vi "fpga_main.vi"() -> ()   [LabVIEW 2013]
uses:
  <vilib>/rvi/FXPMathLib/FxpDiv/subVIs/nifxpmath_Div_SimConfig.ctl
  <vilib>/rvi/Emulation/niFpgaSctlEmulationGetInTimedLoop.vi
  <vilib>/rvi/eio/common/nirviEmuTemplateMethod_errors.vi
  <vilib>/rvi/Emulation/niFpgaProcessEmulError.vi
  <vilib>/rvi/Emulation/niFpgaEmulationReportErrorSimple.vi
  <vilib>/rvi/Emulation/niFpgaGetClockAttributes.vi
  <vilib>/rvi/FXPMathLib/FxpDiv/simVIs/DllFxpDivTemp_sub.vi
  <vilib>/rvi/Emulation/niFpgaCriticalErrorInLSC.vi
  <vilib>/rvi/interface/RandomDataEmulation/nirviRandomDataFPGAFIFO.vi
  <vilib>/rvi/interface/RandomDataEmulation/niFpgaRandomDataHandleErrors.vi
  <vilib>/eio/EIONode/EIONode.xnode
  <vilib>/rvi/FXPMathLib/FxpDiv/XNode/nifxpmath_Div.xnode
  <vilib>/rvi/FXPMathLib/FxpMul/XNode/nifxpmath_Multiplier.xnode
  <vilib>/rvi/FXPMathLib/FxpSub/XNode/nifxpmath_Sub.xnode
  <vilib>/rvi/FXPMathLib/FxpAdd/XNode/nifxpmath_Add.xnode
  <vilib>/rvi/DataTransferAndStorage/Container/XNode/niFpgaContainer.xnode
  <vilib>/rvi/interface/RandomDataEmulation/nirviRandomDataFpgaReadWriteTemplate.vi
  <vilib>/rvi/FXPMathLib/sim/FxpSim.dll
panel:
  out "CoinToss":bool
  out "AutoDispense 4":bool
  out "AutoDispense 3":bool
  out "AutoDispense 1":bool
  out "AutoDispense 2":bool
  out "SensorOffset 4":bool
  out "SensorOffset 3":bool
  out "SensorOffset 2":bool
  out "SensorOffset 1":bool
  in  "Opto On Time 1 (mSec)":u32=5000
  out "Opto Rand Pre":bool
  out "OptoPre 4":bool
  out "OptoPre 3":bool
  out "OptoPre 2":bool
  out "npcountout 4":i16
  in  "npcountin 4":i16
  out "npcountout 3":i16
  in  "npcountin 3":i16
  out "npcountout 2":i16
  in  "npcountin 2":i16
  out "npcountout":i16
  in  "npcountin":i16
  out "angle_out 4":bool
  out "angle_out 3":bool
  out "angle_out 2":bool
  out "angle_out 1":bool
  out "Contingency 4":bool
  out "AI9":fxp<+/-,24,5>
  out "AI8":fxp<+/-,24,5>
  out "Contingency 3":bool
  out "AI6":fxp<+/-,24,5>
  out "AI5":fxp<+/-,24,5>
  out "Contingency 2":bool
  out "AI4":fxp<+/-,24,5>
  out "AI3":fxp<+/-,24,5>
  out "Contingency 1":bool
  out "AI1":fxp<+/-,24,5>
  out "AI2":fxp<+/-,24,5>
  out "flashdisp 4":bool
  out "flashdisp 3":bool
  out "flashdisp 2":bool
  out "flashdisp 1":bool
  out "Automatic Dispense Trigger 4":bool
  out "Automatic Dispense Trigger 3":bool
  in  "Trial Live In 1":bool
  in  "Hold In 1":bool
  in  "Hold Count In 1":i16 format="%.0g"
  out "TurnOnOpto 1":bool
  out "Dispense Trigger 1":bool
  in  "Trial Live In 4":bool
  in  "Hold In 4":bool
  in  "Hold Count In 4":i16 format="%.0g"
  out "TurnOnOpto 4":bool
  out "Opto Rand Met 1":bool
  out "Opto Rand Met 4":bool
  out "Dispense Trigger 4":bool
  in  "Trial Live In 3":bool
  in  "Hold In 3":bool
  in  "Hold Count In 3":i16 format="%.0g"
  in  "Trial Live In 2":bool
  in  "Hold In 2":bool
  in  "Hold Count In 2":i16 format="%.0g"
  out "Opto Rand Met 3":bool
  out "Opto Rand Met 2":bool
  out "TurnOnOpto 3":bool
  out "TurnOnOpto 2":bool
  out "Automatic Dispense Trigger 2":bool
  out "Dispense Trigger 3":bool
  out "Dispense Trigger 2":bool
  out "Automatic Dispense Trigger 1":bool
  in  "Tab Control":T1(tab)
  in  "Automated Pellets Target 1":u16=200
  in  "X Center 1":fxp<+/-,24,5>
  in  "Y Center 1":fxp<+/-,24,5>
  in  "Radius Voltage 1":fxp<+/-,24,5>=1.0
  out "Touch 1 1":bool
  out "Touch 2 1":bool
  out "Nose Poke 1":bool
  out "X 1":fxp<+/-,22,10> format="%.16g"
  out "Y 1":fxp<+/-,22,10> format="%.16g"
  in  "Inner Threshold 1":fxp<+,22,9>=100.0 format="%.23g"
  in  "Hold Duration 1":i16=50
  out "Trial Live 1":bool
  out "Hold 1":bool
  out "Hold Count 1":i16 format="%.0g"
  out "Deviation 1":fxp<+,22,10> format="%.16g"
  in  "Sequence Override 1":bool
  in  "OptoEnable 1":bool
  out "Automated Pellets Dispensed 1":u16
  out "Pellets Dispensed 1":u16
  out "Dispense 1":bool
  in  "Automatic Dispense 1":bool
  in  "Mean 1":fxp<+,22,9>=100.0
  in  "Opto Chance 1 %":fxp<+,16,8>=50.0
  out "Lick 1":bool
  in  "Override Fail when moved out":bool
  in  "Dispense time 1":u32=100
  out "angle":fxp<+/-,9,9>
  in  "Flip 1 1":bool
  in  "Flip 2 1":bool
  in  "Flip XY 1":bool
  in  "Outer\nThreshold 1":fxp<+,22,9>=1.0
  in  "Min Angle 1":fxp<+,9,9> format="%.52g"
  in  "Max Angle 1":fxp<+,9,9>=360.0 format="%.52g"
  in  "Override Approach 1":bool
  in  "Opto on 1":bool
  in  "CCW(T) 1":bool
  in  "Min Angle 1 2":fxp<+,9,9> format="%.52g"
  in  "Max Angle 1 2":fxp<+,9,9>=360.0 format="%.52g"
  in  "CCW(T) 1 2":bool
  in  "Opto OnPost Time 1 (mSec)":u32=5000
  in  "Opto on 2":bool
  out "Deviation 2":fxp<+,22,10> format="%.16g"
  in  "Inner Threshold 2":fxp<+,22,9>=100.0 format="%.23g"
  in  "Hold Duration 2":i16=50
  out "Trial Live 2":bool
  out "Hold 2":bool
  out "Hold Count 2":i16 format="%.0g"
  out "Automated Pellets Dispensed 2":u16
  in  "Automated Pellets Target 2":u16
  out "Pellets Dispensed 2":u16
  in  "Automatic Dispense 2":bool
  in  "Mean 2":fxp<+,22,9>=100.0
  out "Dispense 2":bool
  out "Y 2":fxp<+/-,22,10> format="%.16g"
  out "X 2":fxp<+/-,22,10> format="%.16g"
  out "Nose Poke 2":bool
  out "Touch 2 2":bool
  out "Touch 1 2":bool
  in  "Radius Voltage 2":fxp<+/-,24,5>=1.0
  in  "Flip XY 2":bool
  in  "Flip 2 2":bool
  in  "Flip 1 2":bool
  in  "Outer\nThreshold 2":fxp<+,22,9>=1.0
  in  "Y Center 2":fxp<+/-,24,5>
  in  "X Center 2":fxp<+/-,24,5>
  in  "Sequence Override 2":bool
  in  "OptoEnable 2":bool
  in  "Opto Chance 2 %":fxp<+,16,8>=50.0
  out "Lick 2":bool
  in  "Override Fail when moved out 2":bool
  in  "Dispense time 2":u32=100
  out "angle 2":fxp<+/-,9,9>
  in  "Opto On Time 2 (mSec)":u32=5000
  in  "Override Approach 2":bool
  in  "Min Angle 2":fxp<+,9,9> format="%.52g"
  in  "Max Angle 2":fxp<+,9,9>=360.0 format="%.52g"
  in  "CCW(T)  2":bool
  in  "CCW(T)  2 2":bool
  in  "Min Angle 2 2":fxp<+,9,9> format="%.52g"
  in  "Max Angle 2 2":fxp<+,9,9>=360.0 format="%.52g"
  in  "Opto OnPost Time 2 (mSec)":u32=5000
  out "Deviation 3":fxp<+,22,10> format="%.16g"
  in  "Inner Threshold 3":fxp<+,22,9>=100.0 format="%.23g"
  in  "Hold Duration 3":i16=50
  out "Hold 3":bool
  out "Hold Count 3":i16 format="%.0g"
  out "Trial Live 3":bool
  out "Y 3":fxp<+/-,22,10> format="%.16g"
  out "X 3":fxp<+/-,22,10> format="%.16g"
  out "Nose Poke 3":bool
  out "Touch 2 3":bool
  out "Touch 1 3":bool
  in  "Radius Voltage 3":fxp<+/-,24,5>=1.0
  in  "Flip XY 3":bool
  in  "Flip 2 3":bool
  in  "Flip 1 3":bool
  in  "Outer\nThreshold 3":fxp<+,22,9>=1.0
  in  "Y Center 3":fxp<+/-,24,5>
  in  "X Center 3":fxp<+/-,24,5>
  out "Dispense 3":bool
  in  "Automatic Dispense 3":bool
  in  "Mean 3":fxp<+,22,9>=100.0
  out "Pellets Dispensed 3":u16
  in  "Automated Pellets Target 3":u16
  out "Automated Pellets Dispensed 3":u16
  in  "Sequence Override 3":bool
  in  "OptoEnable 3":bool
  in  "Opto On Time 3(mSec)":u32=5000 caption="Opto On Time 3 (mSec)"
  in  "Opto Chance 3 %":fxp<+,16,8>=50.0
  out "Lick 3":bool
  in  "Override Fail when moved out 3":bool
  in  "Dispense time 3":u32=100
  out "angle 3":fxp<+/-,9,9>
  in  "Override Approach 3":bool
  in  "Opto on 3":bool
  in  "Min Angle 3":fxp<+,9,9> format="%.52g"
  in  "Max Angle 3":fxp<+,9,9>=360.0 format="%.52g"
  in  "CCW(T)  3":bool
  in  "Min Angle 3 2":fxp<+,9,9> format="%.52g"
  in  "Max Angle 3 2":fxp<+,9,9>=360.0 format="%.52g"
  in  "CCW(T)  3 2":bool
  in  "Opto OnPost Time 3 (mSec)":u32=5000
  in  "Opto On Time 4 (mSec)":u32=5000
  in  "X Center 4":fxp<+/-,24,5>
  in  "Y Center 4":fxp<+/-,24,5>
  in  "Outer\nThreshold 4":fxp<+,22,9>=1.0
  in  "Flip 1 4":bool
  in  "Flip 2 4":bool
  in  "Flip XY 4":bool
  in  "Radius Voltage 4":fxp<+/-,24,5>=1.0
  out "Touch 1 4":bool
  out "Touch 2 4":bool
  out "Nose Poke 4":bool
  out "X 4":fxp<+/-,22,10> format="%.16g"
  out "Y 4":fxp<+/-,22,10> format="%.16g"
  in  "Inner Threshold 4":fxp<+,22,9>=100.0 format="%.23g"
  in  "Hold Duration 4":i16=50
  out "Hold 4":bool
  out "Hold Count 4":i16 format="%.0g"
  out "Trial Live 4":bool
  out "Deviation 4":fxp<+,22,10> format="%.16g"
  in  "Sequence Override 4":bool
  in  "OptoEnable 4":bool
  out "Automated Pellets Dispensed 4":u16
  out "Pellets Dispensed 4":u16
  in  "Automated Pellets Target 4":u16
  out "Dispense 4":bool
  in  "Automatic Dispense 4":bool
  in  "Mean 4":fxp<+,22,9>=100.0
  in  "Opto Chance 4 %":fxp<+,16,8>=50.0
  out "Lick 4":bool
  in  "Override Fail when moved out 4":bool
  in  "Dispense time 4":u32=100
  out "angle 4":fxp<+/-,9,9>
  in  "Override Approach 4":bool
  in  "Opto on 4":bool
  in  "Min Angle 4":fxp<+,9,9> format="%.52g"
  in  "Max Angle 4":fxp<+,9,9>=360.0 format="%.52g"
  in  "CCW(T)  4":bool
  in  "Min Angle 4 2":fxp<+,9,9> format="%.52g"
  in  "Max Angle 4 2":fxp<+,9,9>=360.0 format="%.52g"
  in  "CCW(T)  4 2":bool
  in  "Opto OnPost Time 4 (mSec)":u32=5000
  in  "Opto Current 2 (mA)":fxp<+/-,16,8>=65.0
  in  "Opto Offset 2 (mA)":fxp<+/-,16,8>=41.0
  in  "Opto Offset 3 (mA)":fxp<+/-,16,8>=29.0
  in  "Opto Current 3 (mA)":fxp<+/-,16,8>=55.0
  in  "Opto Offset 4 (mA)":fxp<+/-,16,8>=32.0
  in  "Opto Current 4 (mA)":fxp<+/-,16,8>=82.0
  in  "Opto Offset 1 (mA)":fxp<+/-,16,8>
  in  "Opto Current 1 (mA)":fxp<+/-,16,8>
  in  "State Machine States":T2(ring)
  out "ON Duration (usec)":u32
  out "Tick Count(uSec)":u32
  out "Start Tick Count":u32
  out "State Machine States OUT":T2(ring)
  out "Automatic Dispense Trigger 1 Latching":bool
  out "Dispense Trigger 1 Latching":bool
  out "Automatic Dispense Trigger 2 Latching":bool
  out "Dispense Trigger 2 Latching":bool
  out "Automatic Dispense Trigger 3 Latching":bool
  out "Dispense Trigger 3 Latching":bool
  out "Dispense Trigger 4 Latching":bool
  out "Automatic Dispense Trigger 4 Latching":bool
  in  "OptoSeed":u32=4294967295 caption="seed"
  in  "Opto OnPre Time 1 (mSec)":u32=1000
  in  "Opto Chance Pre %":fxp<+,16,8>=2.0
  out "rnd_op":fxp<+,16,1>
  out "fxp_optopre":fxp<+,16,1>
  out "MaskingLightLatch 4":bool
  out "MaskingLightLatch 1":bool
  out "rnd_op 2":fxp<+,16,1>
  out "MaskingLightLatch 2":bool
  out "MaskingLightLatch 3":bool
  in  "Reset Overflow":bool
  out "Proc Time":u32
  out "Overflow":bool
  in  "Acquire Enable":bool
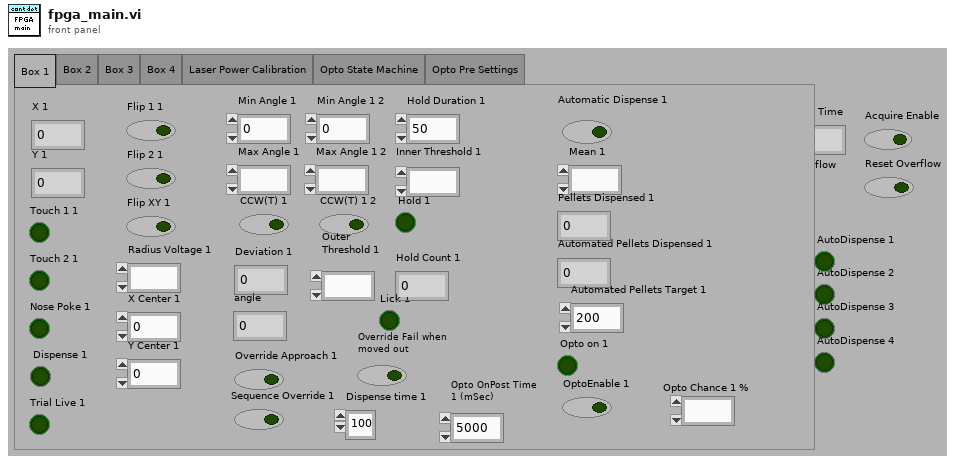
[diagram p1: front panel]
types:
  T1 = enum32{"Box 1", "Box 2", "Box 3", "Box 4", "Laser Power Calibration", "Opto State Machine", "Opto Pre Settings"}
  T2 = enum16{"Listening", "Turn ON", "Timing", "Turn OFF"}
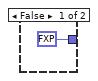
[diagram p2: hidden frame]
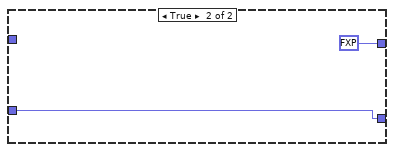
[diagram p3: hidden frame]
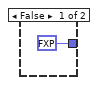
[diagram p4: hidden frame]
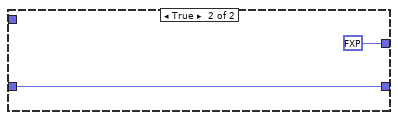
[diagram p5: hidden frame]
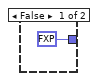
[diagram p6: hidden frame]
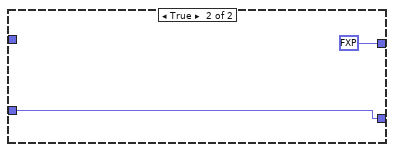
[diagram p7: hidden frame]
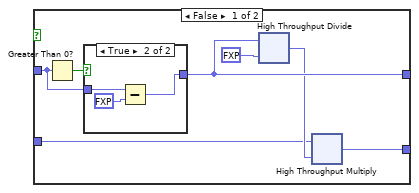
[diagram p10: hidden frame]
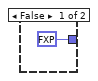
[diagram p11: hidden frame]
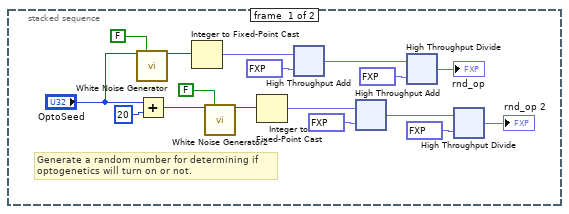
[diagram p14: hidden frame]
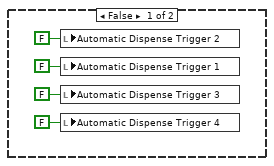
[diagram p15: hidden frame]
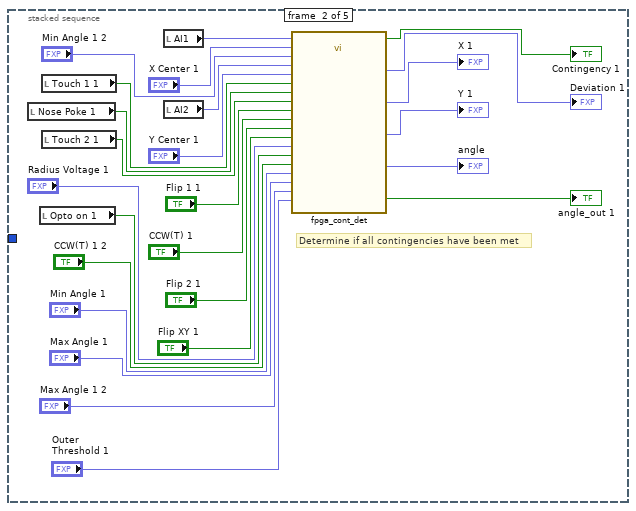
[diagram p16: hidden frame]
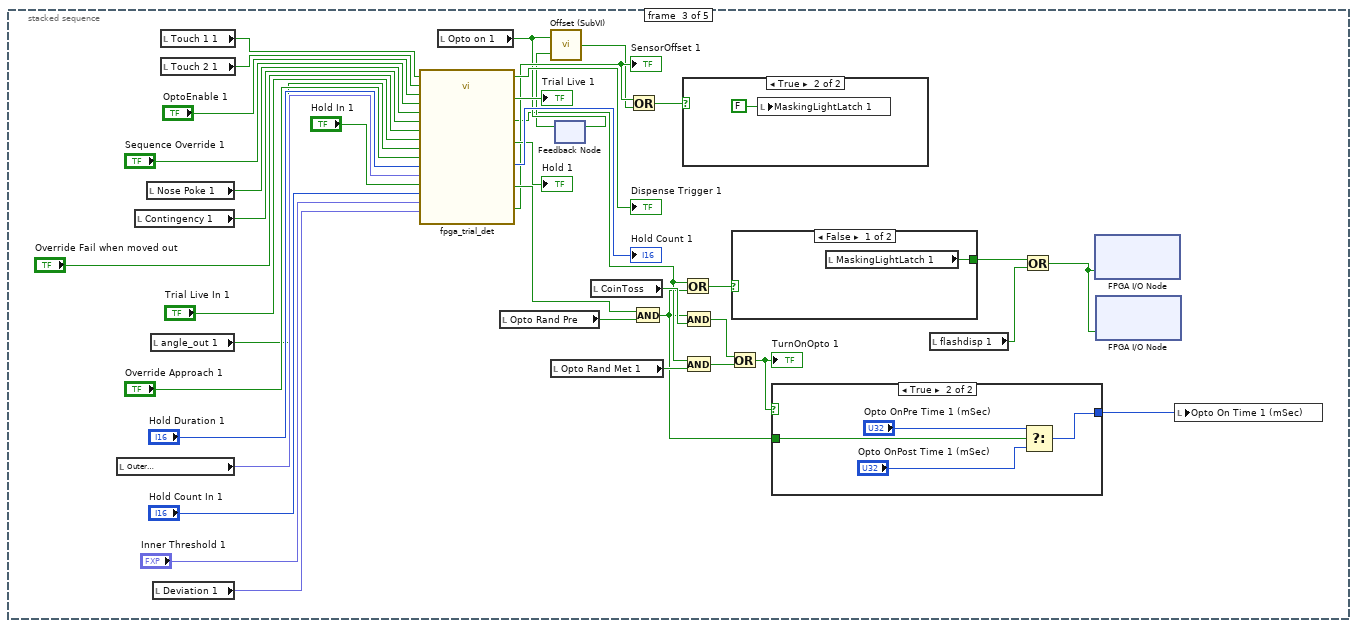
[diagram p17: hidden frame]
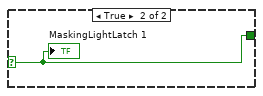
[diagram p19: hidden frame]
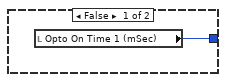
[diagram p20: hidden frame]
diagram:
  w2 = i16 0 ("Hold Count 1")
  w3 = FALSE ("Automatic Dispense Trigger 1 Latching")
  # "FPGA Pinout:\nAI0\nAI1\nAI2\nAI3\nAI4\nAI5\nAI6\nAI7\nAI8\nAI9\nAI10\nAI11\nAI12\nAI13\nAI14\nAI15\nAO"
  n1 = local write "Automatic Dispense Trigger 1 Latching"(w3) -> ()
  n2 = local write "Automatic Dispense Trigger 2 Latching"(w3) -> ()
  n3 = local write "Automatic Dispense Trigger 3 Latching"(w3) -> ()
  n4 = local write "Automatic Dispense Trigger 4 Latching"(w3) -> ()
  n5 = while {
    shift-right: [w37] -> _
    shift-left: _ -> [w36]
    stop <- FALSE stop-if-true
    # "Box 1 Opto On"
    n6 = flat-sequence {
      tunnel: w36 -> [w39]
      tunnel: [w39] -> w35
      tunnel: [w41] -> w37
      tunnel: w35 -> [w59]
      frame #0 {
        n7 = call "Loop Timer13"("Count(uSec)"=u32 1000) -> ()  [unwired: 1 out]
      }
      frame #1 {
        w66 = fxp<+/-,16,16> 32767.0 ("y")
        n8 = xnode "High Throughput Subtract"("x"="Opto Current 1 (mA)", "y"="Opto Offset 1 (mA)") -> ("x-y"=w55:fxp<+/-,17,9>)
        n9 = xnode "High Throughput Divide"("x"=w55, "y"="Opto Current 1 (mA)") -> ("x/y"=w54:fxp<+/-,17,3>)
        n10 = xnode ("High Throughput Multiply")("x"=w54, "y"=fxp<+/-,16,2> 1.25) -> ("x*y"=w52:fxp<+/-,16,8>)
        n11 = case shown="False" "Opto on 1" {
          tunnel: [w122 w161] -> w58
          tunnel: w52 -> [w123 w161]
          tunnel: [w126 fxp<+/-,16,8> 100.0 ("x-y")] -> w41
          tunnel: w59 -> [w127 _]
          frame False {
            n12 = Greater Than 0?(x=w127) -> (x > 0?=w128:bool)
            n13 = case shown="True" w128 {
              tunnel: w127 -> [_ w158]
              tunnel: [fxp<+/-,16,8> 0.0 w157] -> w126
              frame False {
              }
              frame True {
                n14 = Subtract(x=w158, y=fxp<+/-,16,8> 1.0) -> (x-y=w157:fxp<+/-,16,8>)
              }
            }
            n15 = xnode "High Throughput Divide"("x"=w126, "y"=fxp<+/-,16,16> 100.0) -> ("x/y"=w124:fxp<+/-,16,8>)
            n16 = xnode ("High Throughput Multiply")("x"=w123, "y"=w124) -> ("x*y"=w122:fxp<+/-,16,8>)
          }
          frame True {
          }
        }
        n17 = feedback #1() -> (w61:bool)  [unwired: 1 in]
        n18 = Not(x=w61) -> (.not. x?=w62:bool)
        n19 = feedback-in #1("Opto on 1") -> ()
        n20 = And(x=w62, y="Opto on 1") -> (x .and. y?=w60:bool)
        n21 = call "Sine Wave Generator4"("reset"=w60) -> ("sine out"=w65:i16)  [unwired: 14 in]
        n22 = Integer to Fixed-Point Cast(fixed-point type=w66, integer=w65) -> (fixed-point=w67:fxp<+/-,16,16>)
        n23 = xnode "High Throughput Divide"("x"="Opto Offset 1 (mA)", "y"="Opto Current 1 (mA)") -> ("x/y"=w49:fxp<+/-,16,8>)
        n24 = xnode "High Throughput Divide"("x"=w67, "y"=w66) -> ("x/y"=w64:fxp<+/-,16,8>)
        n25 = Greater Than 0?(x=w41) -> (x > 0?=w44:bool)
        n26 = xnode ("High Throughput Multiply")("x"=w64, "y"=w58) -> ("x*y"=w63:fxp<+/-,16,8>)
        n27 = xnode ("High Throughput Multiply")("x"=w49, "y"=fxp<+/-,16,3> 2.5) -> ("x*y"=w47:fxp<+/-,16,8>)
        n28 = Boolean To (0,1)(Boolean=w44) -> (0, 1=w45:i16)
        n29 = xnode ("High Throughput Add")("x"=w63, "y"=w58) -> ("x+y"=w56:fxp<+/-,16,8>)
        n30 = xnode ("High Throughput Add")("x"=w56, "y"=w47) -> ("x+y"=w42:fxp<+/-,16,8>)
        n31 = Integer to Fixed-Point Cast(integer=w45) -> (fixed-point=w46:fxp<+/-,16,16>)  [unwired: 1 in]
        n32 = xnode ("High Throughput Multiply")("x"=w42, "y"=w46) -> ("x*y"=w43:fxp<+/-,16,8>)
        n33 = xnode "FPGA I/O Node"("AO3"=w43) -> ()  [unwired: 1 in, 1 out]
      }
    }
  }
  n34 = local write "Dispense Trigger 1 Latching"(w3) -> ()
  n35 = local write "Dispense Trigger 2 Latching"(w3) -> ()
  n36 = local write "Dispense Trigger 3 Latching"(w3) -> ()
  n37 = local write "Dispense Trigger 4 Latching"(w3) -> ()
  n38 = local write "flashdisp 1"(FALSE ("flashdisp 1")) -> ()
  n39 = local write "flashdisp 2"(FALSE ("flashdisp 2")) -> ()
  n40 = local write "flashdisp 3"(FALSE ("flashdisp 3")) -> ()
  n41 = local write "flashdisp 4"(FALSE ("flashdisp 4")) -> ()
  n42 = while {
    shift-right: [w190] -> _
    shift-left: u16 0 -> [w192]
    stop <- FALSE stop-if-true
    # "Box 2 Dispense"
    n43 = flat-sequence {
      tunnel: w192 -> [w195]
      tunnel: [w195] -> w191
      tunnel: w191 -> [w205]
      tunnel: [w204] -> w190
      tunnel: [w198] -> w189
      frame #0 {
        n44 = call "Loop Timer2"("Count(uSec)"=u32 1000) -> ()  [unwired: 1 out]
      }
      frame #1 {
        n45 = local read "Automatic Dispense Trigger 2 Latching"() -> (w199:bool)
        n46 = local read "Automated Pellets Dispensed 2"() -> (w197:u16)
        n47 = local read "Dispense Trigger 2 Latching"() -> (w200:bool)
        n48 = Less?(x=w197, y="Automated Pellets Target 2") -> (x < y?=w202:bool)
        n49 = And(x=w202, y=w199) -> (x .and. y?=w196:bool)
        n50 = Or(x=w200, y=w196) -> (x .or. y?=w203:bool)
        n51 = case shown="True" w203 {
          tunnel: w205 -> [w207 w215]
          tunnel: [w207 w214] -> w204
          tunnel: w197 -> [w206 w210]
          tunnel: [w206 w213] -> w198
          tunnel: w196 -> [_ w208]
          frame False {
          }
          frame True {
            n52 = flat-sequence {
              tunnel: w215 -> [w218]
              tunnel: [w218] -> w212
              tunnel: [w217] -> w211
              tunnel: w210 -> [w217]
              tunnel: [w216] -> w209
              tunnel: w208 -> [w216]
              tunnel: [w230] -> w213
              tunnel: [w232] -> w214
              tunnel: w212 -> [w233]
              tunnel: w211 -> [w229]
              tunnel: w209 -> [w231]
              frame #0 {
                n53 = flat-sequence {
                  tunnel: w216 -> [w224]
                  frame #0 {
                    w225 = TRUE ("Port0/DIO3")
                    n54 = xnode "FPGA I/O Node"("DIO16"=w225) -> ()  [unwired: 1 in, 1 out]
                    "Dispense 2" <- w225
                    "AutoDispense 2" <- w224
                  }
                  frame #1 {
                    n55 = call "Wait"("Count(mSec)"="Dispense time 2") -> ()  [unwired: 1 out]
                  }
                  frame #2 {
                    w227 = FALSE
                    n56 = local write "AutoDispense 2"(w227) -> ()
                    n57 = local write "Dispense 2"(w227) -> ()
                    n58 = xnode "FPGA I/O Node"("DIO16"=w227) -> ()  [unwired: 1 in, 1 out]
                  }
                }
                n59 = for {
                  N: 2 -> [_]
                  n60 = flat-sequence {
                    frame #0 {
                      "flashdisp 2" <- TRUE ("flasdisp 1")
                    }
                    frame #1 {
                      n61 = call "Wait12"("Count(mSec)"=u32 100) -> ()  [unwired: 1 out]
                    }
                    frame #2 {
                      n62 = local write "flashdisp 2"(FALSE ("flashdisp 1")) -> ()
                    }
                    frame #3 {
                      n63 = call "Wait13"("Count(mSec)"=u32 100) -> ()  [unwired: 1 out]
                    }
                  }
                }
              }
              frame #1 {
                w234 = FALSE ("Automatic Dispense Trigger 2 Latching")
                n64 = Boolean To (0,1)(Boolean=w231) -> (0, 1=w228:i16)
                n65 = local write "Automatic Dispense Trigger 2 Latching"(w234) -> ()
                n66 = local write "Dispense Trigger 2 Latching"(w234) -> ()
                n67 = Add(x=w229, y=w228) -> (x+y=w230:u16)
                n68 = Increment(x=w233) -> (x+1=w232:u16)
              }
            }
          }
        }
      }
    }
    "Pellets Dispensed 2" <- w190
    "Automated Pellets Dispensed 2" <- w189
  }
  n69 = while {
    shift-right: [w236] -> _
    shift-left: u16 0 -> [w237]
    stop <- FALSE stop-if-true
    # "Box 1 Dispense"
    n70 = flat-sequence {
      tunnel: [w240] -> w238
      tunnel: w237 -> [w240]
      tunnel: [w251] -> w236
      tunnel: w238 -> [w248]
      tunnel: [w243] -> w235
      frame #0 {
        n71 = call "Loop Timer9"("Count(uSec)"=u32 1000) -> ()  [unwired: 1 out]
      }
      frame #1 {
        n72 = local read "Automatic Dispense Trigger 1 Latching"() -> (w245:bool)
        n73 = local read "Automated Pellets Dispensed 1"() -> (w244:u16)
        n74 = local read "Dispense Trigger 1 Latching"() -> (w250:bool)
        n75 = Less?(x=w244, y="Automated Pellets Target 1") -> (x < y?=w246:bool)
        n76 = And(x=w246, y=w245) -> (x .and. y?=w242:bool)
        n77 = Or(x=w250, y=w242) -> (x .or. y?=w249:bool)
        n78 = case shown="True" w249 {
          tunnel: w248 -> [w253 w258]
          tunnel: [w253 w259] -> w251
          tunnel: w242 -> [_ w261]
          tunnel: w244 -> [w252 w257]
          tunnel: [w252 w260] -> w243
          frame False {
          }
          frame True {
            n79 = flat-sequence {
              tunnel: w261 -> [w262]
              tunnel: w258 -> [w263]
              tunnel: w257 -> [w264]
              tunnel: [w262] -> w256
              tunnel: [w264] -> w255
              tunnel: [w263] -> w254
              tunnel: [w276] -> w259
              tunnel: [w275] -> w260
              tunnel: w256 -> [w279]
              tunnel: w255 -> [w278]
              tunnel: w254 -> [w277]
              frame #0 {
                n80 = flat-sequence {
                  tunnel: w262 -> [w270]
                  frame #0 {
                    w271 = TRUE ("Port0/DIO3")
                    n81 = xnode "FPGA I/O Node"("DIO23"=w271) -> ()  [unwired: 1 in, 1 out]
                    "Dispense 1" <- w271
                    "AutoDispense 1" <- w270
                  }
                  frame #1 {
                    n82 = call "Wait8"("Count(mSec)"="Dispense time 1") -> ()  [unwired: 1 out]
                  }
                  frame #2 {
                    w273 = FALSE
                    n83 = local write "AutoDispense 1"(w273) -> ()
                    n84 = local write "Dispense 1"(w273) -> ()
                    n85 = xnode "FPGA I/O Node"("DIO23"=w273) -> ()  [unwired: 1 in, 1 out]
                  }
                }
                n86 = for {
                  N: 2 -> [_]
                  n87 = flat-sequence {
                    frame #0 {
                      "flashdisp 1" <- TRUE ("flasdisp 1")
                    }
                    frame #1 {
                      n88 = call "Wait9"("Count(mSec)"=u32 100) -> ()  [unwired: 1 out]
                    }
                    frame #2 {
                      n89 = local write "flashdisp 1"(FALSE ("flashdisp 1")) -> ()
                    }
                    frame #3 {
                      n90 = call "Wait10"("Count(mSec)"=u32 100) -> ()  [unwired: 1 out]
                    }
                  }
                }
              }
              frame #1 {
                w280 = FALSE ("Automatic Dispense Trigger 1 Latching")
                n91 = Boolean To (0,1)(Boolean=w279) -> (0, 1=w274:i16)
                n92 = local write "Automatic Dispense Trigger 1 Latching"(w280) -> ()
                n93 = local write "Dispense Trigger 1 Latching"(w280) -> ()
                n94 = Add(x=w278, y=w274) -> (x+y=w275:u16)
                n95 = Increment(x=w277) -> (x+1=w276:u16)
              }
            }
          }
        }
      }
    }
    "Pellets Dispensed 1" <- w236
    "Automated Pellets Dispensed 1" <- w235
  }
  n96 = while {
    shift-right: [w282] -> _
    shift-left: u16 0 -> [w283]
    stop <- FALSE stop-if-true
    # "Box 3 Dispense"
    n97 = flat-sequence {
      tunnel: [w286] -> w284
      tunnel: w283 -> [w286]
      tunnel: w284 -> [w295]
      tunnel: [w294] -> w282
      tunnel: [w290] -> w281
      frame #0 {
        n98 = call "Loop Timer3"("Count(uSec)"=u32 1000) -> ()  [unwired: 1 out]
      }
      frame #1 {
        n99 = local read "Automatic Dispense Trigger 3 Latching"() -> (w291:bool)
        n100 = local read "Automated Pellets Dispensed 3"() -> (w289:u16)
        n101 = local read "Dispense Trigger 3 Latching"() -> (w297:bool)
        n102 = Less?(x=w289, y="Automated Pellets Target 3") -> (x < y?=w292:bool)
        n103 = And(x=w292, y=w291) -> (x .and. y?=w288:bool)
        n104 = Or(x=w297, y=w288) -> (x .or. y?=w296:bool)
        n105 = case shown="True" w296 {
          tunnel: w295 -> [w299 w306]
          tunnel: [w299 w307] -> w294
          tunnel: w288 -> [_ w300]
          tunnel: w289 -> [w298 w305]
          tunnel: [w298 w301] -> w290
          frame False {
          }
          frame True {
            n106 = flat-sequence {
              tunnel: w300 -> [w308]
              tunnel: w306 -> [w309]
              tunnel: w305 -> [w310]
              tunnel: [w308] -> w304
              tunnel: [w310] -> w303
              tunnel: [w309] -> w302
              tunnel: [w321] -> w307
              tunnel: w304 -> [w324]
              tunnel: w303 -> [w323]
              tunnel: w302 -> [w322]
              tunnel: [w320] -> w301
              frame #0 {
                n107 = flat-sequence {
                  tunnel: w308 -> [w316]
                  frame #0 {
                    w317 = TRUE ("Port0/DIO3")
                    n108 = xnode "FPGA I/O Node"("DIO9"=w317) -> ()  [unwired: 1 in, 1 out]
                    "Dispense 3" <- w317
                    "AutoDispense 3" <- w316
                  }
                  frame #1 {
                    n109 = call "Wait3"("Count(mSec)"="Dispense time 3") -> ()  [unwired: 1 out]
                  }
                  frame #2 {
                    w319 = FALSE
                    n110 = local write "AutoDispense 3"(w319) -> ()
                    n111 = local write "Dispense 3"(w319) -> ()
                    n112 = xnode "FPGA I/O Node"("DIO9"=w319) -> ()  [unwired: 1 in, 1 out]
                  }
                }
                n113 = for {
                  N: 2 -> [_]
                  n114 = flat-sequence {
                    frame #0 {
                      "flashdisp 3" <- TRUE ("flasdisp 1")
                    }
                    frame #1 {
                      n115 = call "Wait15"("Count(mSec)"=u32 100) -> ()  [unwired: 1 out]
                    }
                    frame #2 {
                      n116 = local write "flashdisp 3"(FALSE ("flashdisp 1")) -> ()
                    }
                    frame #3 {
                      n117 = call "Wait16"("Count(mSec)"=u32 100) -> ()  [unwired: 1 out]
                    }
                  }
                }
              }
              frame #1 {
                w326 = FALSE ("Automatic Dispense Trigger 3 Latching")
                n118 = Boolean To (0,1)(Boolean=w324) -> (0, 1=w325:i16)
                n119 = local write "Automatic Dispense Trigger 3 Latching"(w326) -> ()
                n120 = local write "Dispense Trigger 3 Latching"(w326) -> ()
                n121 = Add(x=w323, y=w325) -> (x+y=w320:u16)
                n122 = Increment(x=w322) -> (x+1=w321:u16)
              }
            }
          }
        }
      }
    }
    "Pellets Dispensed 3" <- w282
    "Automated Pellets Dispensed 3" <- w281
  }
  n123 = while {
    shift-right: [w328] -> _
    shift-left: u16 0 -> [w329]
    stop <- FALSE stop-if-true
    # "Box 4 Dispense"
    n124 = flat-sequence {
      tunnel: [w332] -> w330
      tunnel: w329 -> [w332]
      tunnel: w330 -> [w341]
      tunnel: [w340] -> w328
      tunnel: [w337] -> w327
      frame #0 {
        n125 = call "Loop Timer8"("Count(uSec)"=u32 1000) -> ()  [unwired: 1 out]
      }
      frame #1 {
        n126 = local read "Automatic Dispense Trigger 4 Latching"() -> (w335:bool)
        n127 = local read "Automated Pellets Dispensed 4"() -> (w336:u16)
        n128 = local read "Dispense Trigger 4 Latching"() -> (w343:bool)
        n129 = Less?(x=w336, y="Automated Pellets Target 4") -> (x < y?=w338:bool)
        n130 = And(x=w338, y=w335) -> (x .and. y?=w334:bool)
        n131 = Or(x=w343, y=w334) -> (x .or. y?=w342:bool)
        n132 = case shown="True" w342 {
          tunnel: w341 -> [w345 w350]
          tunnel: [w345 w353] -> w340
          tunnel: w334 -> [_ w352]
          tunnel: w336 -> [w344 w346]
          tunnel: [w344 w348] -> w337
          frame False {
          }
          frame True {
            n133 = flat-sequence {
              tunnel: w352 -> [w354]
              tunnel: [w354] -> w351
              tunnel: w350 -> [w356]
              tunnel: [w356] -> w349
              tunnel: w346 -> [w355]
              tunnel: [w355] -> w347
              tunnel: [w370] -> w353
              tunnel: w351 -> [w369]
              tunnel: w349 -> [w368]
              tunnel: [w367] -> w348
              tunnel: w347 -> [w366]
              frame #0 {
                n134 = flat-sequence {
                  tunnel: w354 -> [w362]
                  frame #0 {
                    w363 = TRUE ("Port0/DIO3")
                    n135 = xnode "FPGA I/O Node"("DIO2"=w363) -> ()  [unwired: 1 in, 1 out]
                    "Dispense 4" <- w363
                    "AutoDispense 4" <- w362
                  }
                  frame #1 {
                    n136 = call "Wait7"("Count(mSec)"="Dispense time 4") -> ()  [unwired: 1 out]
                  }
                  frame #2 {
                    w365 = FALSE
                    n137 = local write "AutoDispense 4"(w365) -> ()
                    n138 = local write "Dispense 4"(w365) -> ()
                    n139 = xnode "FPGA I/O Node"("DIO2"=w365) -> ()  [unwired: 1 in, 1 out]
                  }
                }
                n140 = for {
                  N: 2 -> [_]
                  n141 = flat-sequence {
                    frame #0 {
                      "flashdisp 4" <- TRUE ("flasdisp 1")
                    }
                    frame #1 {
                      n142 = call "Wait18"("Count(mSec)"=u32 100) -> ()  [unwired: 1 out]
                    }
                    frame #2 {
                      n143 = local write "flashdisp 4"(FALSE ("flashdisp 1")) -> ()
                    }
                    frame #3 {
                      n144 = call "Wait19"("Count(mSec)"=u32 100) -> ()  [unwired: 1 out]
                    }
                  }
                }
              }
              frame #1 {
                w372 = FALSE ("Automatic Dispense Trigger 4 Latching")
                n145 = Boolean To (0,1)(Boolean=w369) -> (0, 1=w371:i16)
                n146 = local write "Automatic Dispense Trigger 4 Latching"(w372) -> ()
                n147 = local write "Dispense Trigger 4 Latching"(w372) -> ()
                n148 = Add(x=w366, y=w371) -> (x+y=w367:u16)
                n149 = Increment(x=w368) -> (x+1=w370:u16)
              }
            }
          }
        }
      }
    }
    "Pellets Dispensed 4" <- w328
    "Automated Pellets Dispensed 4" <- w327
  }
  n150 = while {
    shift-right: [w375] -> _
    shift-left: fxp<+/-,16,8> 0.0 ("x-y") -> [w374]
    stop <- FALSE stop-if-true
    # "Box 2 Opto On"
    n151 = flat-sequence {
      tunnel: w374 -> [w377]
      tunnel: [w377] -> w373
      tunnel: [w379] -> w375
      tunnel: w373 -> [w397]
      frame #0 {
        n152 = call "Loop Timer10"("Count(uSec)"=u32 1000) -> ()  [unwired: 1 out]
      }
      frame #1 {
        w404 = fxp<+/-,16,16> 32767.0 ("y")
        n153 = xnode "High Throughput Subtract"("x"="Opto Current 2 (mA)", "y"="Opto Offset 2 (mA)") -> ("x-y"=w393:fxp<+/-,17,9>)
        n154 = xnode "High Throughput Divide"("x"=w393, "y"="Opto Current 2 (mA)") -> ("x/y"=w392:fxp<+/-,17,3>)
        n155 = xnode ("High Throughput Multiply")("x"=w392, "y"=fxp<+/-,16,2> 1.25) -> ("x*y"=w390:fxp<+/-,16,8>)
        n156 = case shown="True" "Opto on 2" {
          tunnel: [w460 w499] -> w396
          tunnel: w390 -> [w461 w499]
          tunnel: [w464 fxp<+/-,16,8> 100.0 ("x-y")] -> w379
          tunnel: w397 -> [w465 _]
          frame False {
            n157 = Greater Than 0?(x=w465) -> (x > 0?=w466:bool)
            n158 = case shown="True" w466 {
              tunnel: w465 -> [_ w496]
              tunnel: [fxp<+/-,16,8> 0.0 w495] -> w464
              frame False {
              }
              frame True {
                n159 = Subtract(x=w496, y=fxp<+/-,16,8> 1.0) -> (x-y=w495:fxp<+/-,16,8>)
              }
            }
            n160 = xnode "High Throughput Divide"("x"=w464, "y"=fxp<+/-,16,16> 100.0) -> ("x/y"=w462:fxp<+/-,16,8>)
            n161 = xnode ("High Throughput Multiply")("x"=w461, "y"=w462) -> ("x*y"=w460:fxp<+/-,16,8>)
          }
          frame True {
          }
        }
        n162 = feedback #2() -> (w399:bool)  [unwired: 1 in]
        n163 = Not(x=w399) -> (.not. x?=w400:bool)
        n164 = feedback-in #2("Opto on 2") -> ()
        n165 = And(x=w400, y="Opto on 2") -> (x .and. y?=w398:bool)
        n166 = call "Sine Wave Generator"("reset"=w398) -> ("sine out"=w403:i16)  [unwired: 14 in]
        n167 = Integer to Fixed-Point Cast(fixed-point type=w404, integer=w403) -> (fixed-point=w405:fxp<+/-,16,16>)
        n168 = xnode "High Throughput Divide"("x"="Opto Offset 2 (mA)", "y"="Opto Current 2 (mA)") -> ("x/y"=w387:fxp<+/-,16,8>)
        n169 = xnode "High Throughput Divide"("x"=w405, "y"=w404) -> ("x/y"=w402:fxp<+/-,16,8>)
        n170 = Greater Than 0?(x=w379) -> (x > 0?=w382:bool)
        n171 = xnode ("High Throughput Multiply")("x"=w402, "y"=w396) -> ("x*y"=w401:fxp<+/-,16,8>)
        n172 = xnode ("High Throughput Multiply")("x"=w387, "y"=fxp<+/-,16,3> 2.5) -> ("x*y"=w385:fxp<+/-,16,8>)
        n173 = Boolean To (0,1)(Boolean=w382) -> (0, 1=w383:i16)
        n174 = xnode ("High Throughput Add")("x"=w401, "y"=w396) -> ("x+y"=w394:fxp<+/-,16,8>)
        n175 = xnode ("High Throughput Add")("x"=w394, "y"=w385) -> ("x+y"=w381:fxp<+/-,16,8>)
        n176 = Integer to Fixed-Point Cast(integer=w383) -> (fixed-point=w384:fxp<+/-,16,16>)  [unwired: 1 in]
        n177 = xnode ("High Throughput Multiply")("x"=w381, "y"=w384) -> ("x*y"=w380:fxp<+/-,16,8>)
        n178 = xnode "FPGA I/O Node"("AO2"=w380) -> ()  [unwired: 1 in, 1 out]
      }
    }
  }
  n179 = while {
    shift-right: [w529] -> _
    shift-left: fxp<+/-,16,8> 0.0 ("x-y") -> [w528]
    stop <- FALSE stop-if-true
    # "Box 3 Opto On"
    n180 = flat-sequence {
      tunnel: w528 -> [w531]
      tunnel: [w531] -> w527
      tunnel: [w533] -> w529
      tunnel: w527 -> [w551]
      frame #0 {
        n181 = call "Loop Timer11"("Count(uSec)"=u32 1000) -> ()  [unwired: 1 out]
      }
      frame #1 {
        w558 = fxp<+/-,16,16> 32767.0 ("y")
        n182 = xnode "High Throughput Subtract"("x"="Opto Current 3 (mA)", "y"="Opto Offset 3 (mA)") -> ("x-y"=w547:fxp<+/-,17,9>)
        n183 = xnode "High Throughput Divide"("x"=w547, "y"="Opto Current 3 (mA)") -> ("x/y"=w546:fxp<+/-,17,3>)
        n184 = xnode ("High Throughput Multiply")("x"=w546, "y"=fxp<+/-,16,2> 1.25) -> ("x*y"=w544:fxp<+/-,16,8>)
        n185 = case shown="False" "Opto on 3" {
          tunnel: [w614 w653] -> w550
          tunnel: w544 -> [w615 w653]
          tunnel: [w618 fxp<+/-,16,8> 100.0 ("x-y")] -> w533
          tunnel: w551 -> [w619 _]
          frame False {
            n186 = Greater Than 0?(x=w619) -> (x > 0?=w620:bool)
            n187 = case shown="True" w620 {
              tunnel: w619 -> [_ w650]
              tunnel: [fxp<+/-,16,8> 0.0 w649] -> w618
              frame False {
              }
              frame True {
                n188 = Subtract(x=w650, y=fxp<+/-,16,8> 1.0) -> (x-y=w649:fxp<+/-,16,8>)
              }
            }
            n189 = xnode "High Throughput Divide"("x"=w618, "y"=fxp<+/-,16,16> 100.0) -> ("x/y"=w616:fxp<+/-,16,8>)
            n190 = xnode ("High Throughput Multiply")("x"=w615, "y"=w616) -> ("x*y"=w614:fxp<+/-,16,8>)
          }
          frame True {
          }
        }
        n191 = feedback #3() -> (w553:bool)  [unwired: 1 in]
        n192 = Not(x=w553) -> (.not. x?=w554:bool)
        n193 = feedback-in #3("Opto on 3") -> ()
        n194 = And(x=w554, y="Opto on 3") -> (x .and. y?=w552:bool)
        n195 = call "Sine Wave Generator2"("reset"=w552) -> ("sine out"=w557:i16)  [unwired: 14 in]
        n196 = Integer to Fixed-Point Cast(fixed-point type=w558, integer=w557) -> (fixed-point=w559:fxp<+/-,16,16>)
        n197 = xnode "High Throughput Divide"("x"="Opto Offset 3 (mA)", "y"="Opto Current 3 (mA)") -> ("x/y"=w541:fxp<+/-,16,8>)
        n198 = xnode "High Throughput Divide"("x"=w559, "y"=w558) -> ("x/y"=w556:fxp<+/-,16,8>)
        n199 = Greater Than 0?(x=w533) -> (x > 0?=w537:bool)
        n200 = xnode ("High Throughput Multiply")("x"=w556, "y"=w550) -> ("x*y"=w555:fxp<+/-,16,8>)
        n201 = xnode ("High Throughput Multiply")("x"=w541, "y"=fxp<+/-,16,3> 2.5) -> ("x*y"=w539:fxp<+/-,16,8>)
        n202 = Boolean To (0,1)(Boolean=w537) -> (0, 1=w536:i16)
        n203 = xnode ("High Throughput Add")("x"=w555, "y"=w550) -> ("x+y"=w548:fxp<+/-,16,8>)
        n204 = xnode ("High Throughput Add")("x"=w548, "y"=w539) -> ("x+y"=w534:fxp<+/-,16,8>)
        n205 = Integer to Fixed-Point Cast(integer=w536) -> (fixed-point=w535:fxp<+/-,16,16>)  [unwired: 1 in]
        n206 = xnode ("High Throughput Multiply")("x"=w534, "y"=w535) -> ("x*y"=w538:fxp<+/-,16,8>)
        n207 = xnode "FPGA I/O Node"("AO1"=w538) -> ()  [unwired: 1 in, 1 out]
      }
    }
  }
  n208 = while {
    shift-right: [w683] -> _
    shift-left: fxp<+/-,16,8> 0.0 ("x-y") -> [w682]
    stop <- FALSE stop-if-true
    # "Box 4 Opto On"
    n209 = flat-sequence {
      tunnel: w682 -> [w685]
      tunnel: [w685] -> w681
      tunnel: [w692] -> w683
      tunnel: w681 -> [w710]
      frame #0 {
        n210 = call "Loop Timer12"("Count(uSec)"=u32 1000) -> ()  [unwired: 1 out]
      }
      frame #1 {
        w690 = fxp<+/-,16,16> 32767.0 ("y")
        n211 = xnode "High Throughput Subtract"("x"="Opto Current 4 (mA)", "y"="Opto Offset 4 (mA)") -> ("x-y"=w706:fxp<+/-,17,9>)
        n212 = xnode "High Throughput Divide"("x"=w706, "y"="Opto Current 4 (mA)") -> ("x/y"=w705:fxp<+/-,17,3>)
        n213 = xnode ("High Throughput Multiply")("x"=w705, "y"=fxp<+/-,16,2> 1.25) -> ("x*y"=w703:fxp<+/-,16,8>)
        n214 = case shown="False" "Opto on 4" {
          tunnel: [w795 w834] -> w709
          tunnel: w703 -> [w796 w834]
          tunnel: [w799 fxp<+/-,16,8> 100.0 ("x-y")] -> w692
          tunnel: w710 -> [w800 _]
          frame False {
            n215 = Greater Than 0?(x=w800) -> (x > 0?=w801:bool)
            n216 = case shown="True" w801 {
              tunnel: w800 -> [_ w831]
              tunnel: [fxp<+/-,16,8> 0.0 w830] -> w799
              frame False {
              }
              frame True {
                n217 = Subtract(x=w831, y=fxp<+/-,16,8> 1.0) -> (x-y=w830:fxp<+/-,16,8>)
              }
            }
            n218 = xnode "High Throughput Divide"("x"=w799, "y"=fxp<+/-,16,16> 100.0) -> ("x/y"=w797:fxp<+/-,16,8>)
            n219 = xnode ("High Throughput Multiply")("x"=w796, "y"=w797) -> ("x*y"=w795:fxp<+/-,16,8>)
          }
          frame True {
          }
        }
        n220 = feedback #4() -> (w711:bool)  [unwired: 1 in]
        n221 = Not(x=w711) -> (.not. x?=w712:bool)
        n222 = feedback-in #4("Opto on 4") -> ()
        n223 = And(x=w712, y="Opto on 4") -> (x .and. y?=w687:bool)
        n224 = call "Sine Wave Generator3"("reset"=w687) -> ("sine out"=w689:i16)  [unwired: 14 in]
        n225 = Integer to Fixed-Point Cast(fixed-point type=w690, integer=w689) -> (fixed-point=w691:fxp<+/-,16,16>)
        n226 = xnode "High Throughput Divide"("x"="Opto Offset 4 (mA)", "y"="Opto Current 4 (mA)") -> ("x/y"=w700:fxp<+/-,16,8>)
        n227 = xnode "High Throughput Divide"("x"=w691, "y"=w690) -> ("x/y"=w688:fxp<+/-,16,8>)
        n228 = Greater Than 0?(x=w692) -> (x > 0?=w693:bool)
        n229 = xnode ("High Throughput Multiply")("x"=w688, "y"=w709) -> ("x*y"=w713:fxp<+/-,16,8>)
        n230 = xnode ("High Throughput Multiply")("x"=w700, "y"=fxp<+/-,16,3> 2.5) -> ("x*y"=w695:fxp<+/-,16,8>)
        n231 = Boolean To (0,1)(Boolean=w693) -> (0, 1=w694:i16)
        n232 = xnode ("High Throughput Add")("x"=w713, "y"=w709) -> ("x+y"=w707:fxp<+/-,16,8>)
        n233 = xnode ("High Throughput Add")("x"=w707, "y"=w695) -> ("x+y"=w697:fxp<+/-,16,8>)
        n234 = Integer to Fixed-Point Cast(integer=w694) -> (fixed-point=w696:fxp<+/-,16,16>)  [unwired: 1 in]
        n235 = xnode ("High Throughput Multiply")("x"=w697, "y"=w696) -> ("x*y"=w698:fxp<+/-,16,8>)
        n236 = xnode "FPGA I/O Node"("AO0"=w698) -> ()  [unwired: 1 in, 1 out]
      }
    }
  }
  n237 = xnode "FPGA I/O Node"("DIO16"=FALSE ("DIO14")) -> ()  [unwired: 1 in, 1 out]
  n238 = xnode "FPGA I/O Node"("DIO23"=FALSE ("DIO14")) -> ()  [unwired: 1 in, 1 out]
  n239 = xnode "FPGA I/O Node"("DIO7"=FALSE ("DIO14")) -> ()  [unwired: 1 in, 1 out]
  n240 = xnode "FPGA I/O Node"("DIO9"=FALSE ("DIO14")) -> ()  [unwired: 1 in, 1 out]
  n241 = xnode "FPGA I/O Node"("DIO21"=FALSE ("DIO14")) -> ()  [unwired: 1 in, 1 out]
  n242 = xnode "FPGA I/O Node"("DIO2"=FALSE ("DIO14")) -> ()  [unwired: 1 in, 1 out]
  n243 = xnode "FPGA I/O Node"("DIO0"=FALSE ("DIO14")) -> ()  [unwired: 1 in, 1 out]
  n244 = xnode "FPGA I/O Node"("DIO14"=FALSE) -> ()  [unwired: 1 in, 1 out]
  n245 = while {
    shift-right: [w885] -> _
    shift-left: FALSE -> [w872]
    shift-right: [w866] -> _
    shift-left: FALSE ("Trial Live Out") -> [w881]
    shift-right: [w867] -> _
    shift-left: FALSE ("Trial Live Out") -> [w878]
    shift-right: [w868] -> _
    shift-left: FALSE ("Hold Out") -> [w871]
    shift-right: [w865] -> _
    shift-left: i16 0 ("Hold Count Out") -> [w877]
    shift-right: [w870] -> _
    shift-left: FALSE ("Hold Out") -> [w876]
    shift-right: [w869] -> _
    shift-left: i16 0 ("Hold Count Out") -> [w875]
    shift-right: [w850] -> _
    shift-left: FALSE ("Trial Live 4") -> [w853]
    shift-right: [w852] -> _
    shift-left: FALSE ("Hold 4") -> [w855]
    shift-right: [w851] -> _
    shift-left: i16 0 ("Hold Count 4") -> [w854]
    shift-right: [w846] -> _
    shift-left: FALSE ("TurnOnOpto 3") -> [w849]
    shift-right: [w845] -> _
    shift-left: FALSE ("Hold 1") -> [w848]
    shift-right: [w844] -> _
    shift-left: i16 0 ("Hold Count 1") -> [w847]
    shift-right: [w835] -> _
    shift-left: w2 -> [w842]
    shift-right: [w836] -> _
    shift-left: w2 -> [w839]
    shift-right: [w837] -> _
    shift-left: w2 -> [w840]
    shift-right: [w838] -> _
    shift-left: w2 -> [w841]
    stop <- FALSE stop-if-true
    n246 = flat-sequence {
      tunnel: w881 -> [w904]
      tunnel: w878 -> [w900]
      tunnel: w871 -> [w899]
      tunnel: w877 -> [w901]
      tunnel: w876 -> [w903]
      tunnel: w875 -> [w902]
      tunnel: w855 -> [w898]
      tunnel: w853 -> [w897]
      tunnel: w854 -> [w896]
      tunnel: w849 -> [w895]
      tunnel: w848 -> [w894]
      tunnel: w847 -> [w893]
      tunnel: w842 -> [w889]
      tunnel: w841 -> [w892]
      tunnel: w840 -> [w891]
      tunnel: w839 -> [w890]
      tunnel: [w906] -> w884
      tunnel: [w909] -> w882
      tunnel: w884 -> [w908]
      tunnel: [w908] -> w883
      tunnel: w872 -> [w907]
      tunnel: w883 -> [w916]
      tunnel: [w916] -> w864
      tunnel: w882 -> [w915]
      tunnel: [w915] -> w862
      tunnel: w864 -> [w1167]
      tunnel: [w1167] -> w863
      tunnel: w862 -> [w1169]
      tunnel: [w1169] -> w861
      tunnel: [w1168] -> w843
      tunnel: w863 -> [w1290]
      tunnel: [w1290] -> w880
      tunnel: w861 -> [w1292]
      tunnel: [w1292] -> w879
      tunnel: [w1291] -> w874
      tunnel: [w1410] -> w860
      tunnel: [w1411] -> w858
      tunnel: w879 -> [w1411]
      tunnel: w880 -> [w1410]
      tunnel: [w1412] -> w873
      tunnel: w860 -> [w1530]
      tunnel: [w1530] -> w859
      tunnel: w858 -> [w1532]
      tunnel: [w1532] -> w857
      tunnel: [w1531] -> w856
      tunnel: w859 -> [w1658]
      tunnel: [w1658] -> w887
      tunnel: w857 -> [w1656]
      tunnel: [w1655] -> w886
      tunnel: w874 -> [w1653]
      tunnel: w873 -> [w1652]
      tunnel: w856 -> [w1651]
      tunnel: w843 -> [w1650]
      tunnel: w887 -> [w1686]
      tunnel: [w1684] -> w885
      tunnel: w886 -> [w1684]
      tunnel: [w1683] -> w870
      tunnel: [w1682] -> w869
      tunnel: [w1680] -> w868
      tunnel: [w1679] -> w867
      tunnel: [w1678] -> w866
      tunnel: [w1681] -> w865
      tunnel: [w1677] -> w852
      tunnel: [w1676] -> w851
      tunnel: [w1675] -> w850
      tunnel: [w1674] -> w846
      tunnel: [w1672] -> w845
      tunnel: [w1673] -> w844
      tunnel: [w1671] -> w838
      tunnel: [w1670] -> w837
      tunnel: [w1669] -> w836
      tunnel: [w1668] -> w835
      frame #0 {
        # "1. Start Loop"
        n247 = local write "Hold In 2"(w903) -> ()
        n248 = local write "Hold Count In 2"(w902) -> ()
        n249 = local write "Hold In 4"(w898) -> ()
        n250 = local write "Hold Count In 4"(w896) -> ()
        n251 = local write "Trial Live In 2"(w904) -> ()
        n252 = local write "Trial Live In 3"(w900) -> ()
        n253 = local write "Hold In 3"(w899) -> ()
        n254 = local write "Hold Count In 3"(w901) -> ()
        n255 = local write "Trial Live In 1"(w895) -> ()
        n256 = local write "Hold In 1"(w894) -> ()
        n257 = local write "Hold Count In 1"(w893) -> ()
        n258 = local write "npcountin"(w889) -> ()
        n259 = local write "npcountin 2"(w890) -> ()
        n260 = local write "npcountin 3"(w891) -> ()
        n261 = local write "npcountin 4"(w892) -> ()
        n262 = call "Loop Timer"("Count(uSec)"=u32 1000) -> ()  [unwired: 1 out]
        n263 = local write "Trial Live In 4"(w897) -> ()
      }
      frame #1 {
        # "2. Start Proc Timer"
        n264 = call "Tick Count"() -> ("Tick Count(uSec)"=w906:u32)
      }
      frame #2 {
        # "3. Reset Overflow"
        n265 = Not(x="Reset Overflow") -> (.not. x?=w910:bool)
        n266 = And(x=w907, y=w910) -> (x .and. y?=w909:bool)
      }
      frame #3 {
        # "Determine optogenetic activation:\n0. Generate random numbers\n1. Use random numbers to determine if optogenetics will activate"
        # "4. Automatic Dispensing"
        n267 = stacked-sequence {
          frame #0 {
            # "Generate a random number for determining if \noptogenetics will turn on or not."
            n268 = call "White Noise Generator"("seed"="OptoSeed", "reset"=FALSE) -> ("white noise out"=w930:i16)  [unwired: 13 in]
            n269 = Add(x="OptoSeed", y=u32 20) -> (x+y=w919:u32)
            n270 = Integer to Fixed-Point Cast(integer=w930) -> (fixed-point=w931:fxp<+/-,16,16>)  [unwired: 1 in]
            n271 = call "White Noise Generator2"("seed"=w919, "reset"=FALSE) -> ("white noise out"=w921:i16)  [unwired: 13 in]
            n272 = Integer to Fixed-Point Cast(integer=w921) -> (fixed-point=w925:fxp<+/-,16,16>)  [unwired: 1 in]
            n273 = xnode ("High Throughput Add")("x"=w931, "y"=fxp<+,16,16> 32768.0) -> ("x+y"=w932:fxp<+,18,18>)
            n274 = xnode ("High Throughput Add")("x"=w925, "y"=fxp<+,16,16> 32768.0) -> ("x+y"=w926:fxp<+,18,18>)
            n275 = xnode "High Throughput Divide"("x"=w932, "y"=fxp<+,18,18> 65536.0) -> ("x/y"=→"rnd_op":fxp<+,16,1>)
            n276 = xnode "High Throughput Divide"("x"=w926, "y"=fxp<+,18,18> 65536.0) -> ("x/y"=→"rnd_op 2":fxp<+,16,1>)
          }
          frame #1 {
            n277 = local read "rnd_op 2"() -> (w990:fxp<+,16,1>)
            n278 = Less Or Equal?(x=w990, y=fxp<+,16,1> 0.5) -> (x <= y?=→"CoinToss":bool)
            n279 = xnode "High Throughput Divide"("x"="Opto Chance 2 %", "y"=fxp<+,16,16> 100.0) -> ("x/y"=w1015:fxp<+,16,1>)
            n280 = xnode "High Throughput Divide"("x"="Opto Chance Pre %", "y"=fxp<+,16,16> 100.0) -> ("x/y"=w994:fxp<+,16,1>)
            "fxp_optopre" <- w994
            n281 = xnode "High Throughput Divide"("x"="Opto Chance 1 %", "y"=fxp<+,16,16> 100.0) -> ("x/y"=w997:fxp<+,16,1>)
            n282 = xnode "High Throughput Divide"("x"="Opto Chance 4 %", "y"=fxp<+,16,16> 100.0) -> ("x/y"=w1009:fxp<+,16,1>)
            n283 = xnode "High Throughput Divide"("x"="Opto Chance 3 %", "y"=fxp<+,16,16> 100.0) -> ("x/y"=w1005:fxp<+,16,1>)
            n284 = local read "rnd_op"() -> (w1011:fxp<+,16,1>)
            n285 = local read "rnd_op"() -> (w992:fxp<+,16,1>)
            n286 = local read "rnd_op"() -> (w996:fxp<+,16,1>)
            n287 = local read "rnd_op"() -> (w1006:fxp<+,16,1>)
            n288 = local read "rnd_op"() -> (w1001:fxp<+,16,1>)
            n289 = Less Or Equal?(x=w1011, y=w1015) -> (x <= y?=→"Opto Rand Met 2":bool)
            n290 = Less Or Equal?(x=w992, y=w994) -> (x <= y?=→"Opto Rand Pre":bool)
            n291 = Less Or Equal?(x=w996, y=w997) -> (x <= y?=→"Opto Rand Met 1":bool)
            n292 = Less Or Equal?(x=w1006, y=w1009) -> (x <= y?=→"Opto Rand Met 4":bool)
            n293 = Less Or Equal?(x=w1001, y=w1005) -> (x <= y?=→"Opto Rand Met 3":bool)
          }
        }
        n294 = xnode ("FIFO Method Node")() -> ("Number of Elements to Read"=w914:u32)  [unwired: 1 in, 1 out]
        n295 = Greater Than 0?(x=w914) -> (x > 0?=w913:bool)
        n296 = To Long Integer(number=w914) -> (32bit integer=w912:i32)
        n297 = case shown="True" w913 {
          tunnel: w912 -> [_ w1155]
          frame False {
            n298 = local write "Automatic Dispense Trigger 2"(FALSE ("Automatic Dispense Trigger")) -> ()
            n299 = local write "Automatic Dispense Trigger 1"(FALSE ("Automatic Dispense Trigger")) -> ()
            n300 = local write "Automatic Dispense Trigger 3"(FALSE ("Automatic Dispense Trigger 3")) -> ()
            n301 = local write "Automatic Dispense Trigger 4"(FALSE ("Automatic Dispense Trigger 4")) -> ()
          }
          frame True {
            n302 = for {
              N: w1155 -> [_]
              n303 = xnode ("FIFO Method Node")("Timeout"=0) -> ("Element"=w1165:u8)  [unwired: 1 in, 2 out]
              n304 = Number To Boolean Array(number=w1165) -> (Boolean array=w1163:bool[])
              n305 = Index Array(array=w1163, index #1=0 ("index"), index #2=1 ("index"), index #3=2 ("index"), index #4=3 ("index")) -> (element #1=→"Automatic Dispense Trigger 1":bool, element #2=→"Automatic Dispense Trigger 2":bool, element #3=→"Automatic Dispense Trigger 3":bool, element #4=→"Automatic Dispense Trigger 4":bool)
            }
          }
        }
      }
      frame #4 {
        n306 = stacked-sequence {
          tunnel: [_ _ _ _ w1283] -> w1168
          tunnel: w1167 -> [_ _ _ w1273 _]
          frame #0 {
            n307 = xnode "FPGA I/O Node"() -> ("AI1"=w1185:fxp<+/-,24,5>, "AI2"=w1179:fxp<+/-,24,5>, "DIO25"=w1178:bool, "DIO26"=w1176:bool, "DIO27"=→"Lick 1":bool, "DIO22"=w1172:bool)  [unwired: 6 in, 6 out]
            n308 = feedback #5() -> (w1183:fxp<+/-,24,5>)  [unwired: 1 in]
            n309 = feedback #6() -> (w1181:fxp<+/-,24,5>)  [unwired: 1 in]
            n310 = feedback-in #7(w1185) -> ()
            n311 = feedback #7() -> (w1184:fxp<+/-,24,5>)  [unwired: 1 in]
            n312 = feedback-in #5(w1184) -> ()
            n313 = call "3ptmed.vi"("s2"=w1183, "s1"=w1184, "s0"=w1185) -> ("sout"=→"AI1":fxp<+/-,24,5>)
            n314 = feedback #8() -> (w1182:fxp<+/-,24,5>)  [unwired: 1 in]
            n315 = feedback-in #6(w1182) -> ()
            n316 = call "3ptmed.vi"("s2"=w1181, "s1"=w1182, "s0"=w1179) -> ("sout"=→"AI2":fxp<+/-,24,5>)
            n317 = feedback-in #8(w1179) -> ()
            n318 = call "np_delay_off (SubVI).vi"("Nose poke in"=w1172, "npcountin"="npcountin") -> ("Nose Poke out"=→"Nose Poke 1":bool, "npcountout"=→"npcountout":i16)
            n319 = feedback #9() -> (w1175:bool)  [unwired: 1 in]
            n320 = call "debouncer (SubVI).vi"("Touch in Prev"=w1175, "Touch in"=w1176) -> ("Touch out"=→"Touch 1 1":bool)
            n321 = feedback-in #9(w1176) -> ()
            n322 = feedback #10() -> (w1177:bool)  [unwired: 1 in]
            n323 = call "debouncer (SubVI).vi"("Touch in Prev"=w1177, "Touch in"=w1178) -> ("Touch out"=→"Touch 2 1":bool)
            n324 = feedback-in #10(w1178) -> ()
          }
          frame #1 {
            # "Determine if all contingencies have been met"
            n325 = local read "Nose Poke 1"() -> (w1208:bool)
            n326 = local read "Opto on 1"() -> (w1189:bool)
            n327 = local read "Touch 1 1"() -> (w1209:bool)
            n328 = local read "Touch 2 1"() -> (w1207:bool)
            n329 = local read "AI1"() -> (w1213:fxp<+/-,24,5>)
            n330 = local read "AI2"() -> (w1211:fxp<+/-,24,5>)
            n331 = call "fpga_cont_det.vi"("X"=w1213, "X Center"="X Center 1", "Min Angle 2"="Min Angle 1 2", "Y"=w1211, "Y Center"="Y Center 1", "Touch 1"=w1209, "Nose Poke"=w1208, "Touch 2"=w1207, "Threshold"="Outer\nThreshold 1", "Flip 1"="Flip 1 1", "Max Angle 2"="Max Angle 1 2", "CCW(T)"="CCW(T) 1", "Max Angle"="Max Angle 1", "Flip 2"="Flip 2 1", "Min Angle"="Min Angle 1", "Flip XY"="Flip XY 1", "CCW(T)  2"="CCW(T) 1 2", "Radius Voltage"="Radius Voltage 1", "Laser ?"=w1189) -> ("Contingency"=→"Contingency 1":bool, "Deviation"=→"Deviation 1":fxp<+,22,10>, "X"=→"X 1":fxp<+/-,22,10>, "Y"=→"Y 1":fxp<+/-,22,10>, "angle"=→"angle":fxp<+/-,9,9>, "angle_out"=→"angle_out 1":bool)  [unwired: 3 in]
          }
          frame #2 {
            n332 = local read "Outer\nThreshold 1"() -> (w1233:fxp<+,22,9>)
            n333 = local read "Contingency 1"() -> (w1246:bool)
            n334 = local read "Nose Poke 1"() -> (w1247:bool)
            n335 = local read "angle_out 1"() -> (w1232:bool)
            n336 = local read "Deviation 1"() -> (w1239:fxp<+,22,10>)
            n337 = local read "Touch 1 1"() -> (w1251:bool)
            n338 = local read "Touch 2 1"() -> (w1250:bool)
            n339 = call "fpga_trial_det.vi"("Touch 1"=w1251, "Touch 2"=w1250, "OptoEnable"="OptoEnable 1", "Sequence Override"="Sequence Override 1", "Nose Poke"=w1247, "Contingency"=w1246, "Override Fail when moved out"="Override Fail when moved out", "Trial Live In"="Trial Live In 1", "Deviation"=w1239, "angle_outer"=w1232, "override approach"="Override Approach 1", "Center Hold Threshold"="Inner Threshold 1", "Hold Duration"="Hold Duration 1", "outer threshold"=w1233, "Hold Count In"="Hold Count In 1", "Hold In"="Hold In 1") -> ("Dispense"=→"Dispense Trigger 1":bool, "Trial Live Out"=→"Trial Live 1":bool, "TurnOnOpto"=w1217:bool, "Hold Out"=→"Hold 1":bool, "Hold Count Out"=→"Hold Count 1":i16, "OptoPre"=w1228:bool, "SensorOffset"=w1224:bool)  [unwired: 5 in]
            "SensorOffset 1" <- w1224
            n340 = local read "Opto on 1"() -> (w1222:bool)
            n341 = local read "Opto Rand Pre"() -> (w1227:bool)
            n342 = local read "Opto Rand Met 1"() -> (w1231:bool)
            n343 = feedback #11() -> (w1221:bool)  [unwired: 1 in]
            n344 = call "Offset (SubVI).vi"("bool_in_prev"=w1221, "bool_in"=w1222) -> ("offset"=w1220:bool)
            n345 = feedback-in #11(w1222) -> ()
            n346 = local read "CoinToss"() -> (w1219:bool)
            n347 = Or(x=w1224, y=w1220) -> (x .or. y?=w1223:bool)
            n348 = And(x=w1228, y=w1227) -> (x .and. y?=w1215:bool)
            n349 = case shown="True" w1223 {
              frame False {
              }
              frame True {
                n350 = local write "MaskingLightLatch 1"(FALSE ("MaskingLightLatch 1")) -> ()
              }
            }
            n351 = Or(x=w1217, y=w1215) -> (x .or. y?=w1216:bool)
            n352 = And(x=w1215, y=w1219) -> (x .and. y?=w1218:bool)
            n353 = And(x=w1217, y=w1231) -> (x .and. y?=w1229:bool)
            n354 = Or(x=w1218, y=w1229) -> (x .or. y?=w1226:bool)
            "TurnOnOpto 1" <- w1226
            n355 = case shown="False" w1216 {
              selector: w1216 -> [_ w1255]
              tunnel: [w1254 w1255] -> w1225
              frame False {
                n356 = local read "MaskingLightLatch 1"() -> (w1254:bool)
              }
              frame True {
                "MaskingLightLatch 1" <- w1255
              }
            }
            n357 = case shown="True" w1226 {
              tunnel: w1215 -> [_ w1260]
              tunnel: [w1256 w1258] -> w1230
              frame False {
                n358 = local read "Opto On Time 1 (mSec)"() -> (w1256:u32)
              }
              frame True {
                n359 = Select(t="Opto OnPre Time 1 (mSec)", s=w1260, f="Opto OnPost Time 1 (mSec)") -> (s? t:f=w1258:u32)
              }
            }
            n360 = local read "flashdisp 1"() -> (w1252:bool)
            n361 = Or(x=w1225, y=w1252) -> (x .or. y?=w1214:bool)
            n362 = xnode "FPGA I/O Node"("DIO24"=w1214) -> ()  [unwired: 1 in, 1 out]
            n363 = xnode "FPGA I/O Node"("DIO21"=w1214) -> ()  [unwired: 1 in, 1 out]
            n364 = local write "Opto On Time 1 (mSec)"(w1230) -> ()
          }
          frame #3 {
            n365 = local read "Dispense Trigger 1"() -> (w1263:bool)
            n366 = local read "SensorOffset 1"() -> (w1262:bool)
            n367 = local read "TurnOnOpto 1"() -> (w1270:bool)
            n368 = case shown="True" w1263 {
              frame False {
              }
              frame True {
                "Dispense Trigger 1 Latching" <- TRUE ("Dispense Trigger 1 Latching")
              }
            }
            n369 = Not(x=w1262) -> (.not. x?=w1261:bool)
            n370 = local read "Automatic Dispense Trigger 1"() -> (w1264:bool)
            n371 = call "OptoOnStateMachine_2016_5_31_1654.vi"("Touch 1"=w1261, "State Machine States"="State Machine States", "Opto On Time 1 (mSec)"="Opto On Time 1 (mSec)", "Tick Count(uSec) in"=w1273, "TurnOnOpto 1"=w1270) -> ("Boolean"=w1272:bool, "State Machine States OUT"=→"State Machine States OUT":T2, "Tick Count(uSec) out"=→"Tick Count(uSec)":u32, "Start Tick Count"=→"Start Tick Count":u32, "ON Duration (usec)"=→"ON Duration (usec)":u32)  [unwired: 2 in]
            n372 = local write "Opto on 1"(w1272) -> ()
            n373 = case shown="True" w1264 {
              tunnel: w1264 -> [_ w1275]
              frame False {
              }
              frame True {
                "Automatic Dispense Trigger 1 Latching" <- w1275
              }
            }
          }
          frame #4 {
            n374 = local read "AutoDispense 1"() -> (w1278:bool)
            n375 = local read "Nose Poke 1"() -> (w1281:bool)
            n376 = local read "Dispense 1"() -> (w1285:bool)
            n377 = local read "Trial Live 1"() -> (w1279:bool)
            n378 = local read "Touch 1 1"() -> (w1280:bool)
            n379 = local read "Touch 2 1"() -> (w1282:bool)
            n380 = local read "Opto on 1"() -> (w1286:bool)
            n381 = local read "Lick 1"() -> (w1284:bool)
            n382 = Build Array(w1280, w1282, w1281, w1285, w1286, w1284, w1279, w1278) -> (w1287:bool[])
            n383 = local read "X 1"() -> (w1276:fxp<+/-,22,10>)
            n384 = local read "Y 1"() -> (w1277:fxp<+/-,22,10>)
            n385 = Boolean Array To Number(Boolean array=w1287) -> (number=w1289:u8)
            n386 = Integer to Fixed-Point Cast(fixed-point type=w1277, integer=w1289) -> (fixed-point=w1288:fxp<+/-,22,10>)
            n387 = Build Array(w1276, w1277, w1288) -> (w1283:fxp<+/-,22,10>[])
          }
        }
      }
      frame #5 {
        # "6. Box 2: Acquire, Contingency Detect"
        n388 = stacked-sequence {
          tunnel: [_ _ _ _ w1408] -> w1291
          tunnel: w1290 -> [_ _ _ w1393 _]
          frame #0 {
            n389 = xnode "FPGA I/O Node"() -> ("AI3"=w1307:fxp<+/-,24,5>, "AI4"=w1302:fxp<+/-,24,5>, "DIO18"=w1300:bool, "DIO19"=w1299:bool, "DIO20"=→"Lick 2":bool, "DIO15"=w1295:bool)  [unwired: 6 in, 6 out]
            n390 = feedback #12() -> (w1305:fxp<+/-,24,5>)  [unwired: 1 in]
            n391 = feedback #13() -> (w1309:fxp<+/-,24,5>)  [unwired: 1 in]
            n392 = feedback #14() -> (w1304:fxp<+/-,24,5>)  [unwired: 1 in]
            n393 = feedback-in #12(w1304) -> ()
            n394 = call "3ptmed.vi"("s2"=w1305, "s1"=w1304, "s0"=w1302) -> ("sout"=→"AI4":fxp<+/-,24,5>)
            n395 = feedback-in #14(w1302) -> ()
            n396 = feedback #15() -> (w1308:fxp<+/-,24,5>)  [unwired: 1 in]
            n397 = feedback-in #13(w1308) -> ()
            n398 = call "3ptmed.vi"("s2"=w1309, "s1"=w1308, "s0"=w1307) -> ("sout"=→"AI3":fxp<+/-,24,5>)
            n399 = feedback-in #15(w1307) -> ()
            n400 = call "np_delay_off (SubVI).vi"("Nose poke in"=w1295, "npcountin"="npcountin 2") -> ("Nose Poke out"=→"Nose Poke 2":bool, "npcountout"=→"npcountout 2":i16)
            n401 = feedback #16() -> (w1298:bool)  [unwired: 1 in]
            n402 = call "debouncer (SubVI).vi"("Touch in Prev"=w1298, "Touch in"=w1299) -> ("Touch out"=→"Touch 1 2":bool)
            n403 = feedback-in #16(w1299) -> ()
            n404 = feedback #17() -> (w1301:bool)  [unwired: 1 in]
            n405 = call "debouncer (SubVI).vi"("Touch in Prev"=w1301, "Touch in"=w1300) -> ("Touch out"=→"Touch 2 2":bool)
            n406 = feedback-in #17(w1300) -> ()
          }
          frame #1 {
            n407 = local read "Nose Poke 2"() -> (w1325:bool)
            n408 = local read "Opto on 2"() -> (w1313:bool)
            n409 = local read "Touch 1 2"() -> (w1327:bool)
            n410 = local read "Touch 2 2"() -> (w1326:bool)
            n411 = local read "AI3"() -> (w1336:fxp<+/-,24,5>)
            n412 = local read "AI4"() -> (w1335:fxp<+/-,24,5>)
            n413 = call "fpga_cont_det.vi"("X"=w1336, "X Center"="X Center 2", "Min Angle 2"="Min Angle 2 2", "Y"=w1335, "Y Center"="Y Center 2", "Touch 1"=w1327, "Nose Poke"=w1325, "Touch 2"=w1326, "Threshold"="Outer\nThreshold 2", "Flip 1"="Flip 1 2", "Max Angle 2"="Max Angle 2 2", "CCW(T)"="CCW(T)  2", "Max Angle"="Max Angle 2", "Flip 2"="Flip 2 2", "Min Angle"="Min Angle 2", "Flip XY"="Flip XY 2", "CCW(T)  2"="CCW(T)  2 2", "Radius Voltage"="Radius Voltage 2", "Laser ?"=w1313) -> ("Contingency"=→"Contingency 2":bool, "Deviation"=→"Deviation 2":fxp<+,22,10>, "X"=→"X 2":fxp<+/-,22,10>, "Y"=→"Y 2":fxp<+/-,22,10>, "angle"=→"angle 2":fxp<+/-,9,9>, "angle_out"=→"angle_out 2":bool)  [unwired: 3 in]
          }
          frame #2 {
            n414 = local read "Touch 1 2"() -> (w1355:bool)
            n415 = case shown="False" w1355 {
              frame False {
                n416 = local write "Opto on 2"(FALSE ("Opto on 2")) -> ()
              }
              frame True {
              }
            }
            n417 = local read "Outer\nThreshold 2"() -> (w1357:fxp<+,22,9>)
            n418 = local read "Contingency 2"() -> (w1371:bool)
            n419 = local read "Nose Poke 2"() -> (w1372:bool)
            n420 = local read "angle_out 2"() -> (w1356:bool)
            n421 = local read "Deviation 2"() -> (w1365:fxp<+,22,10>)
            n422 = local read "Touch 1 2"() -> (w1376:bool)
            n423 = local read "Touch 2 2"() -> (w1375:bool)
            n424 = call "fpga_trial_det.vi"("Touch 1"=w1376, "Touch 2"=w1375, "OptoEnable"="OptoEnable 2", "Sequence Override"="Sequence Override 2", "Nose Poke"=w1372, "Contingency"=w1371, "Override Fail when moved out"="Override Fail when moved out 2", "Trial Live In"="Trial Live In 2", "Deviation"=w1365, "angle_outer"=w1356, "override approach"="Override Approach 2", "Center Hold Threshold"="Inner Threshold 2", "Hold Duration"="Hold Duration 2", "outer threshold"=w1357, "Hold Count In"="Hold Count In 2", "Hold In"="Hold In 2") -> ("Dispense"=→"Dispense Trigger 2":bool, "Trial Live Out"=→"Trial Live 2":bool, "TurnOnOpto"=w1344:bool, "Hold Out"=→"Hold 2":bool, "Hold Count Out"=→"Hold Count 2":i16, "OptoPre"=w1353:bool, "SensorOffset"=w1339:bool)  [unwired: 5 in]
            "OptoPre 2" <- w1353
            "SensorOffset 2" <- w1339
            n425 = local read "Opto on 2"() -> (w1340:bool)
            n426 = local read "Opto Rand Pre"() -> (w1352:bool)
            n427 = local read "Opto Rand Met 2"() -> (w1354:bool)
            n428 = feedback #18() -> (w1342:bool)  [unwired: 1 in]
            n429 = call "Offset (SubVI).vi"("bool_in_prev"=w1342, "bool_in"=w1340) -> ("offset"=w1341:bool)
            n430 = feedback-in #18(w1340) -> ()
            n431 = local read "CoinToss"() -> (w1346:bool)
            n432 = Or(x=w1339, y=w1341) -> (x .or. y?=w1338:bool)
            n433 = And(x=w1353, y=w1352) -> (x .and. y?=w1343:bool)
            n434 = case shown="True" w1338 {
              frame False {
              }
              frame True {
                n435 = local write "MaskingLightLatch 2"(FALSE ("MaskingLightLatch 2")) -> ()
              }
            }
            n436 = Or(x=w1344, y=w1343) -> (x .or. y?=w1347:bool)
            n437 = And(x=w1344, y=w1354) -> (x .and. y?=w1351:bool)
            n438 = And(x=w1343, y=w1346) -> (x .and. y?=w1345:bool)
            n439 = case shown="False" w1347 {
              selector: w1347 -> [_ w1379]
              tunnel: [w1378 w1379] -> w1348
              frame False {
                n440 = local read "MaskingLightLatch 2"() -> (w1378:bool)
              }
              frame True {
                "MaskingLightLatch 2" <- w1379
              }
            }
            n441 = Or(x=w1351, y=w1345) -> (x .or. y?=w1350:bool)
            "TurnOnOpto 2" <- w1350
            n442 = case shown="True" w1350 {
              tunnel: [w1380 w1384] -> w1349
              tunnel: w1343 -> [_ w1382]
              frame False {
                n443 = local read "Opto On Time 2 (mSec)"() -> (w1380:u32)
              }
              frame True {
                n444 = local read "Opto OnPre Time 1 (mSec)"() -> (w1383:u32)
                n445 = Select(t=w1383, s=w1382, f="Opto OnPost Time 2 (mSec)") -> (s? t:f=w1384:u32)
              }
            }
            n446 = local read "flashdisp 2"() -> (w1361:bool)
            n447 = Or(x=w1348, y=w1361) -> (x .or. y?=w1337:bool)
            n448 = xnode "FPGA I/O Node"("DIO17"=w1337) -> ()  [unwired: 1 in, 1 out]
            n449 = xnode "FPGA I/O Node"("DIO14"=w1337) -> ()  [unwired: 1 in, 1 out]
            n450 = local write "Opto On Time 2 (mSec)"(w1349) -> ()
          }
          frame #3 {
            n451 = local read "Dispense Trigger 2"() -> (w1389:bool)
            n452 = local read "SensorOffset 2"() -> (w1386:bool)
            n453 = local read "TurnOnOpto 2"() -> (w1392:bool)
            n454 = case shown="True" w1389 {
              tunnel: w1389 -> [_ w1394]
              frame False {
              }
              frame True {
                "Dispense Trigger 2 Latching" <- w1394
              }
            }
            n455 = local read "Automatic Dispense Trigger 2"() -> (w1388:bool)
            n456 = Not(x=w1386) -> (.not. x?=w1387:bool)
            n457 = call "OptoOnStateMachine_2016_5_31_1654.vi"("Touch 1"=w1387, "Opto On Time 1 (mSec)"="Opto On Time 2 (mSec)", "Tick Count(uSec) in"=w1393, "TurnOnOpto 1"=w1392) -> ("Boolean"=w1390:bool)  [unwired: 3 in, 4 out]
            n458 = local write "Opto on 2"(w1390) -> ()
            n459 = case shown="True" w1388 {
              tunnel: w1388 -> [_ w1395]
              frame False {
              }
              frame True {
                "Automatic Dispense Trigger 2 Latching" <- w1395
              }
            }
          }
          frame #4 {
            n460 = local read "AutoDispense 2"() -> (w1396:bool)
            n461 = local read "Nose Poke 2"() -> (w1400:bool)
            n462 = local read "Dispense 2"() -> (w1404:bool)
            n463 = local read "Trial Live 2"() -> (w1397:bool)
            n464 = local read "Touch 1 2"() -> (w1402:bool)
            n465 = local read "Touch 2 2"() -> (w1401:bool)
            n466 = local read "Opto on 2"() -> (w1405:bool)
            n467 = local read "Lick 2"() -> (w1403:bool)
            n468 = Build Array(w1402, w1401, w1400, w1404, w1405, w1403, w1397, w1396) -> (w1407:bool[])
            n469 = local read "Y 2"() -> (w1398:fxp<+/-,22,10>)
            n470 = Boolean Array To Number(Boolean array=w1407) -> (number=w1409:u8)
            n471 = Integer to Fixed-Point Cast(fixed-point type=w1398, integer=w1409) -> (fixed-point=w1406:fxp<+/-,22,10>)
            n472 = local read "X 2"() -> (w1399:fxp<+/-,22,10>)
            n473 = Build Array(w1399, w1398, w1406) -> (w1408:fxp<+/-,22,10>[])
          }
        }
      }
      frame #6 {
        # "7. Box 3: Acquire, Contingency Detect"
        n474 = stacked-sequence {
          tunnel: [_ _ _ _ w1526] -> w1412
          tunnel: w1410 -> [_ _ _ w1512 _]
          frame #0 {
            n475 = xnode "FPGA I/O Node"() -> ("AI5"=w1423:fxp<+/-,24,5>, "AI6"=w1420:fxp<+/-,24,5>, "DIO11"=w1429:bool, "DIO12"=w1427:bool, "DIO13"=→"Lick 3":bool, "DIO8"=w1416:bool)  [unwired: 6 in, 6 out]
            n476 = feedback #19() -> (w1419:fxp<+/-,24,5>)  [unwired: 1 in]
            n477 = feedback #20() -> (w1421:fxp<+/-,24,5>)  [unwired: 1 in]
            n478 = feedback #21() -> (w1418:fxp<+/-,24,5>)  [unwired: 1 in]
            n479 = feedback-in #19(w1418) -> ()
            n480 = call "3ptmed.vi"("s2"=w1419, "s1"=w1418, "s0"=w1420) -> ("sout"=→"AI6":fxp<+/-,24,5>)
            n481 = feedback-in #21(w1420) -> ()
            n482 = feedback #22() -> (w1422:fxp<+/-,24,5>)  [unwired: 1 in]
            n483 = feedback-in #20(w1422) -> ()
            n484 = call "3ptmed.vi"("s2"=w1421, "s1"=w1422, "s0"=w1423) -> ("sout"=→"AI5":fxp<+/-,24,5>)
            n485 = feedback-in #22(w1423) -> ()
            n486 = call "np_delay_off (SubVI).vi"("Nose poke in"=w1416, "npcountin"="npcountin 3") -> ("Nose Poke out"=→"Nose Poke 3":bool, "npcountout"=→"npcountout 3":i16)
            n487 = feedback #23() -> (w1426:bool)  [unwired: 1 in]
            n488 = call "debouncer (SubVI).vi"("Touch in Prev"=w1426, "Touch in"=w1427) -> ("Touch out"=→"Touch 1 3":bool)
            n489 = feedback-in #23(w1427) -> ()
            n490 = feedback #24() -> (w1428:bool)  [unwired: 1 in]
            n491 = call "debouncer (SubVI).vi"("Touch in Prev"=w1428, "Touch in"=w1429) -> ("Touch out"=→"Touch 2 3":bool)
            n492 = feedback-in #24(w1429) -> ()
          }
          frame #1 {
            n493 = local read "Nose Poke 3"() -> (w1447:bool)
            n494 = local read "Opto on 3"() -> (w1432:bool)
            n495 = local read "Touch 1 3"() -> (w1449:bool)
            n496 = local read "Touch 2 3"() -> (w1448:bool)
            n497 = local read "AI5"() -> (w1453:fxp<+/-,24,5>)
            n498 = local read "AI6"() -> (w1451:fxp<+/-,24,5>)
            n499 = call "fpga_cont_det.vi"("X"=w1453, "X Center"="X Center 3", "Min Angle 2"="Min Angle 3 2", "Y"=w1451, "Y Center"="Y Center 3", "Touch 1"=w1449, "Nose Poke"=w1447, "Touch 2"=w1448, "Threshold"="Outer\nThreshold 3", "Flip 1"="Flip 1 3", "Max Angle 2"="Max Angle 3 2", "CCW(T)"="CCW(T)  3", "Max Angle"="Max Angle 3", "Flip 2"="Flip 2 3", "Min Angle"="Min Angle 3", "Flip XY"="Flip XY 3", "CCW(T)  2"="CCW(T)  3 2", "Radius Voltage"="Radius Voltage 3", "Laser ?"=w1432) -> ("Contingency"=→"Contingency 3":bool, "Deviation"=→"Deviation 3":fxp<+,22,10>, "X"=→"X 3":fxp<+/-,22,10>, "Y"=→"Y 3":fxp<+/-,22,10>, "angle"=→"angle 3":fxp<+/-,9,9>, "angle_out"=→"angle_out 3":bool)  [unwired: 3 in]
          }
          frame #2 {
            n500 = local read "Touch 1 3"() -> (w1475:bool)
            n501 = case shown="False" w1475 {
              frame False {
                n502 = local write "Opto on 3"(FALSE ("Opto on 3")) -> ()
              }
              frame True {
              }
            }
            n503 = local read "Outer\nThreshold 3"() -> (w1476:fxp<+,22,9>)
            n504 = local read "Contingency 3"() -> (w1479:bool)
            n505 = local read "Nose Poke 3"() -> (w1491:bool)
            n506 = local read "angle_out 3"() -> (w1477:bool)
            n507 = local read "Deviation 3"() -> (w1484:fxp<+,22,10>)
            n508 = local read "Touch 1 3"() -> (w1495:bool)
            n509 = local read "Touch 2 3"() -> (w1494:bool)
            n510 = call "fpga_trial_det.vi"("Touch 1"=w1495, "Touch 2"=w1494, "OptoEnable"="OptoEnable 3", "Sequence Override"="Sequence Override 3", "Nose Poke"=w1491, "Contingency"=w1479, "Override Fail when moved out"="Override Fail when moved out 3", "Trial Live In"="Trial Live In 3", "Deviation"=w1484, "angle_outer"=w1477, "override approach"="Override Approach 3", "Center Hold Threshold"="Inner Threshold 3", "Hold Duration"="Hold Duration 3", "outer threshold"=w1476, "Hold Count In"="Hold Count In 3", "Hold In"="Hold In 3") -> ("Dispense"=→"Dispense Trigger 3":bool, "Trial Live Out"=→"Trial Live 3":bool, "TurnOnOpto"=w1466:bool, "Hold Out"=→"Hold 3":bool, "Hold Count Out"=→"Hold Count 3":i16, "OptoPre"=w1473:bool, "SensorOffset"=w1459:bool)  [unwired: 5 in]
            "OptoPre 3" <- w1473
            "SensorOffset 3" <- w1459
            n511 = local read "Opto on 3"() -> (w1467:bool)
            n512 = local read "Opto Rand Pre"() -> (w1472:bool)
            n513 = local read "Opto Rand Met 3"() -> (w1474:bool)
            n514 = feedback #25() -> (w1468:bool)  [unwired: 1 in]
            n515 = call "Offset (SubVI).vi"("bool_in_prev"=w1468, "bool_in"=w1467) -> ("offset"=w1461:bool)
            n516 = feedback-in #25(w1467) -> ()
            n517 = local read "CoinToss"() -> (w1462:bool)
            n518 = Or(x=w1459, y=w1461) -> (x .or. y?=w1460:bool)
            n519 = And(x=w1473, y=w1472) -> (x .and. y?=w1463:bool)
            n520 = case shown="True" w1460 {
              frame False {
              }
              frame True {
                n521 = local write "MaskingLightLatch 3"(FALSE ("MaskingLightLatch 3")) -> ()
              }
            }
            n522 = Or(x=w1466, y=w1463) -> (x .or. y?=w1465:bool)
            n523 = And(x=w1466, y=w1474) -> (x .and. y?=w1471:bool)
            n524 = And(x=w1462, y=w1463) -> (x .and. y?=w1464:bool)
            n525 = case shown="True" w1465 {
              selector: w1465 -> [_ w1499]
              tunnel: [w1498 w1499] -> w1458
              frame False {
                n526 = local read "MaskingLightLatch 3"() -> (w1498:bool)
              }
              frame True {
                "MaskingLightLatch 3" <- w1499
              }
            }
            n527 = Or(x=w1471, y=w1464) -> (x .or. y?=w1470:bool)
            "TurnOnOpto 3" <- w1470
            n528 = case shown="True" w1470 {
              tunnel: [w1500 w1502] -> w1469
              tunnel: w1463 -> [_ w1503]
              frame False {
                n529 = local read "Opto On Time 3(mSec)"() -> (w1500:u32)
              }
              frame True {
                n530 = local read "Opto OnPre Time 1 (mSec)"() -> (w1504:u32)
                n531 = Select(t=w1504, s=w1503, f="Opto OnPost Time 3 (mSec)") -> (s? t:f=w1502:u32)
              }
            }
            n532 = local read "flashdisp 3"() -> (w1496:bool)
            n533 = Or(x=w1458, y=w1496) -> (x .or. y?=w1457:bool)
            n534 = xnode "FPGA I/O Node"("DIO10"=w1457) -> ()  [unwired: 1 in, 1 out]
            n535 = xnode "FPGA I/O Node"("DIO7"=w1457) -> ()  [unwired: 1 in, 1 out]
            n536 = local write "Opto On Time 3(mSec)"(w1469) -> ()
          }
          frame #3 {
            n537 = local read "Dispense Trigger 3"() -> (w1508:bool)
            n538 = local read "SensorOffset 3"() -> (w1507:bool)
            n539 = local read "TurnOnOpto 3"() -> (w1513:bool)
            n540 = case shown="True" w1508 {
              tunnel: w1508 -> [_ w1514]
              frame False {
              }
              frame True {
                "Dispense Trigger 3 Latching" <- w1514
              }
            }
            n541 = local read "Automatic Dispense Trigger 3"() -> (w1509:bool)
            n542 = Not(x=w1507) -> (.not. x?=w1506:bool)
            n543 = call "OptoOnStateMachine_2016_5_31_1654.vi"("Touch 1"=w1506, "Opto On Time 1 (mSec)"="Opto On Time 3(mSec)", "Tick Count(uSec) in"=w1512, "TurnOnOpto 1"=w1513) -> ("Boolean"=w1510:bool)  [unwired: 3 in, 4 out]
            n544 = local write "Opto on 3"(w1510) -> ()
            n545 = case shown="True" w1509 {
              tunnel: w1509 -> [_ w1515]
              frame False {
              }
              frame True {
                "Automatic Dispense Trigger 3 Latching" <- w1515
              }
            }
          }
          frame #4 {
            n546 = local read "AutoDispense 3"() -> (w1516:bool)
            n547 = local read "Nose Poke 3"() -> (w1519:bool)
            n548 = local read "Dispense 3"() -> (w1524:bool)
            n549 = local read "Trial Live 3"() -> (w1517:bool)
            n550 = local read "Touch 1 3"() -> (w1521:bool)
            n551 = local read "Touch 2 3"() -> (w1520:bool)
            n552 = local read "Opto on 3"() -> (w1525:bool)
            n553 = local read "Lick 3"() -> (w1518:bool)
            n554 = Build Array(w1521, w1520, w1519, w1524, w1525, w1518, w1517, w1516) -> (w1529:bool[])
            n555 = local read "X 3"() -> (w1522:fxp<+/-,22,10>)
            n556 = Boolean Array To Number(Boolean array=w1529) -> (number=w1528:u8)
            n557 = Integer to Fixed-Point Cast(fixed-point type=w1522, integer=w1528) -> (fixed-point=w1527:fxp<+/-,22,10>)
            n558 = local read "Y 3"() -> (w1523:fxp<+/-,22,10>)
            n559 = Build Array(w1522, w1523, w1527) -> (w1526:fxp<+/-,22,10>[])
          }
        }
      }
      frame #7 {
        # "8. Box 4: Acquire, Contingency Detect"
        n560 = stacked-sequence {
          tunnel: [_ _ _ _ w1646] -> w1531
          tunnel: w1530 -> [_ _ _ w1633 _]
          frame #0 {
            n561 = xnode "FPGA I/O Node"() -> ("AI8"=w1542:fxp<+/-,24,5>, "AI9"=w1538:fxp<+/-,24,5>, "DIO4"=w1549:bool, "DIO5"=w1547:bool, "DIO6"=→"Lick 4":bool, "DIO1"=w1535:bool)  [unwired: 6 in, 6 out]
            n562 = feedback #26() -> (w1541:fxp<+/-,24,5>)  [unwired: 1 in]
            n563 = feedback #27() -> (w1545:fxp<+/-,24,5>)  [unwired: 1 in]
            n564 = feedback #28() -> (w1540:fxp<+/-,24,5>)  [unwired: 1 in]
            n565 = feedback-in #26(w1540) -> ()
            n566 = call "3ptmed.vi"("s2"=w1541, "s1"=w1540, "s0"=w1538) -> ("sout"=→"AI9":fxp<+/-,24,5>)
            n567 = feedback-in #28(w1538) -> ()
            n568 = feedback #29() -> (w1544:fxp<+/-,24,5>)  [unwired: 1 in]
            n569 = feedback-in #27(w1544) -> ()
            n570 = call "3ptmed.vi"("s2"=w1545, "s1"=w1544, "s0"=w1542) -> ("sout"=→"AI8":fxp<+/-,24,5>)
            n571 = feedback-in #29(w1542) -> ()
            n572 = call "np_delay_off (SubVI).vi"("Nose poke in"=w1535, "npcountin"="npcountin 4") -> ("Nose Poke out"=→"Nose Poke 4":bool, "npcountout"=→"npcountout 4":i16)
            n573 = feedback #30() -> (w1546:bool)  [unwired: 1 in]
            n574 = call "debouncer (SubVI).vi"("Touch in Prev"=w1546, "Touch in"=w1547) -> ("Touch out"=→"Touch 1 4":bool)
            n575 = feedback-in #30(w1547) -> ()
            n576 = feedback #31() -> (w1548:bool)  [unwired: 1 in]
            n577 = call "debouncer (SubVI).vi"("Touch in Prev"=w1548, "Touch in"=w1549) -> ("Touch out"=→"Touch 2 4":bool)
            n578 = feedback-in #31(w1549) -> ()
          }
          frame #1 {
            n579 = local read "Nose Poke 4"() -> (w1570:bool)
            n580 = local read "Opto on 4"() -> (w1555:bool)
            n581 = local read "Touch 1 4"() -> (w1572:bool)
            n582 = local read "Touch 2 4"() -> (w1571:bool)
            n583 = local read "AI8"() -> (w1576:fxp<+/-,24,5>)
            n584 = local read "AI9"() -> (w1575:fxp<+/-,24,5>)
            n585 = call "fpga_cont_det.vi"("X"=w1576, "X Center"="X Center 4", "Min Angle 2"="Min Angle 4 2", "Y"=w1575, "Y Center"="Y Center 4", "Touch 1"=w1572, "Nose Poke"=w1570, "Touch 2"=w1571, "Threshold"="Outer\nThreshold 4", "Flip 1"="Flip 1 4", "Max Angle 2"="Max Angle 4 2", "CCW(T)"="CCW(T)  4", "Max Angle"="Max Angle 4", "Flip 2"="Flip 2 4", "Min Angle"="Min Angle 4", "Flip XY"="Flip XY 4", "CCW(T)  2"="CCW(T)  4 2", "Radius Voltage"="Radius Voltage 4", "Laser ?"=w1555) -> ("Contingency"=→"Contingency 4":bool, "Deviation"=→"Deviation 4":fxp<+,22,10>, "X"=→"X 4":fxp<+/-,22,10>, "Y"=→"Y 4":fxp<+/-,22,10>, "angle"=→"angle 4":fxp<+/-,9,9>, "angle_out"=→"angle_out 4":bool)  [unwired: 3 in]
          }
          frame #2 {
            n586 = local read "Touch 1 4"() -> (w1595:bool)
            n587 = case shown="False" w1595 {
              frame False {
                n588 = local write "Opto on 4"(FALSE ("Opto on 4")) -> ()
              }
              frame True {
              }
            }
            n589 = local read "Outer\nThreshold 4"() -> (w1597:fxp<+,22,9>)
            n590 = local read "Contingency 4"() -> (w1610:bool)
            n591 = local read "Nose Poke 4"() -> (w1611:bool)
            n592 = local read "angle_out 4"() -> (w1596:bool)
            n593 = local read "Deviation 4"() -> (w1599:fxp<+,22,10>)
            n594 = local read "Touch 1 4"() -> (w1615:bool)
            n595 = local read "Touch 2 4"() -> (w1614:bool)
            n596 = call "fpga_trial_det.vi"("Touch 1"=w1615, "Touch 2"=w1614, "OptoEnable"="OptoEnable 4", "Sequence Override"="Sequence Override 4", "Nose Poke"=w1611, "Contingency"=w1610, "Override Fail when moved out"="Override Fail when moved out 4", "Trial Live In"="Trial Live In 4", "Deviation"=w1599, "angle_outer"=w1596, "override approach"="Override Approach 4", "Center Hold Threshold"="Inner Threshold 4", "Hold Duration"="Hold Duration 4", "outer threshold"=w1597, "Hold Count In"="Hold Count In 4", "Hold In"="Hold In 4") -> ("Dispense"=→"Dispense Trigger 4":bool, "Trial Live Out"=→"Trial Live 4":bool, "TurnOnOpto"=w1580:bool, "Hold Out"=→"Hold 4":bool, "Hold Count Out"=→"Hold Count 4":i16, "OptoPre"=w1593:bool, "SensorOffset"=w1585:bool)  [unwired: 5 in]
            "OptoPre 4" <- w1593
            "SensorOffset 4" <- w1585
            n597 = local read "Opto on 4"() -> (w1586:bool)
            n598 = local read "Opto Rand Pre"() -> (w1592:bool)
            n599 = local read "Opto Rand Met 4"() -> (w1594:bool)
            n600 = feedback #32() -> (w1587:bool)  [unwired: 1 in]
            n601 = call "Offset (SubVI).vi"("bool_in_prev"=w1587, "bool_in"=w1586) -> ("offset"=w1578:bool)
            n602 = feedback-in #32(w1586) -> ()
            n603 = local read "CoinToss"() -> (w1582:bool)
            n604 = Or(x=w1585, y=w1578) -> (x .or. y?=w1584:bool)
            n605 = And(x=w1593, y=w1592) -> (x .and. y?=w1579:bool)
            n606 = case shown="True" w1584 {
              frame False {
              }
              frame True {
                n607 = local write "MaskingLightLatch 4"(FALSE ("MaskingLightLatch 4")) -> ()
              }
            }
            n608 = Or(x=w1580, y=w1579) -> (x .or. y?=w1581:bool)
            n609 = And(x=w1580, y=w1594) -> (x .and. y?=w1591:bool)
            n610 = And(x=w1579, y=w1582) -> (x .and. y?=w1583:bool)
            n611 = case shown="True" w1581 {
              selector: w1581 -> [_ w1619]
              tunnel: [w1618 w1619] -> w1588
              frame False {
                n612 = local read "MaskingLightLatch 4"() -> (w1618:bool)
              }
              frame True {
                "MaskingLightLatch 4" <- w1619
              }
            }
            n613 = Or(x=w1591, y=w1583) -> (x .or. y?=w1589:bool)
            "TurnOnOpto 4" <- w1589
            n614 = case shown="True" w1589 {
              tunnel: [w1620 w1622] -> w1590
              tunnel: w1579 -> [_ w1621]
              frame False {
                n615 = local read "Opto On Time 4 (mSec)"() -> (w1620:u32)
              }
              frame True {
                n616 = local read "Opto OnPre Time 1 (mSec)"() -> (w1624:u32)
                n617 = Select(t=w1624, s=w1621, f="Opto OnPost Time 4 (mSec)") -> (s? t:f=w1622:u32)
              }
            }
            n618 = local read "flashdisp 4"() -> (w1616:bool)
            n619 = Or(x=w1588, y=w1616) -> (x .or. y?=w1577:bool)
            n620 = xnode "FPGA I/O Node"("DIO3"=w1577) -> ()  [unwired: 1 in, 1 out]
            n621 = xnode "FPGA I/O Node"("DIO0"=w1577) -> ()  [unwired: 1 in, 1 out]
            n622 = local write "Opto On Time 4 (mSec)"(w1590) -> ()
          }
          frame #3 {
            n623 = local read "Dispense Trigger 4"() -> (w1629:bool)
            n624 = local read "SensorOffset 4"() -> (w1626:bool)
            n625 = local read "TurnOnOpto 4"() -> (w1632:bool)
            n626 = local read "Automatic Dispense Trigger 4"() -> (w1628:bool)
            n627 = case shown="True" w1629 {
              tunnel: w1629 -> [_ w1635]
              frame False {
              }
              frame True {
                "Dispense Trigger 4 Latching" <- w1635
              }
            }
            n628 = Not(x=w1626) -> (.not. x?=w1627:bool)
            n629 = call "OptoOnStateMachine_2016_5_31_1654.vi"("Touch 1"=w1627, "Opto On Time 1 (mSec)"="Opto On Time 4 (mSec)", "Tick Count(uSec) in"=w1633, "TurnOnOpto 1"=w1632) -> ("Boolean"=w1630:bool)  [unwired: 3 in, 4 out]
            n630 = local write "Opto on 4"(w1630) -> ()
            n631 = case shown="True" w1628 {
              tunnel: w1628 -> [_ w1634]
              frame False {
              }
              frame True {
                "Automatic Dispense Trigger 4 Latching" <- w1634
              }
            }
          }
          frame #4 {
            n632 = local read "AutoDispense 4"() -> (w1636:bool)
            n633 = local read "Nose Poke 4"() -> (w1643:bool)
            n634 = local read "Dispense 4"() -> (w1642:bool)
            n635 = local read "Trial Live 4"() -> (w1637:bool)
            n636 = local read "Touch 1 4"() -> (w1645:bool)
            n637 = local read "Touch 2 4"() -> (w1644:bool)
            n638 = local read "Opto on 4"() -> (w1641:bool)
            n639 = local read "Lick 4"() -> (w1640:bool)
            n640 = Build Array(w1645, w1644, w1643, w1642, w1641, w1640, w1637, w1636) -> (w1647:bool[])
            n641 = local read "Y 4"() -> (w1638:fxp<+/-,22,10>)
            n642 = Boolean Array To Number(Boolean array=w1647) -> (number=w1649:u8)
            n643 = Integer to Fixed-Point Cast(fixed-point type=w1638, integer=w1649) -> (fixed-point=w1648:fxp<+/-,22,10>)
            n644 = local read "X 4"() -> (w1639:fxp<+/-,22,10>)
            n645 = Build Array(w1639, w1638, w1648) -> (w1646:fxp<+/-,22,10>[])
          }
        }
      }
      frame #8 {
        # "12. FIFO Write"
        n646 = Build Array (concatenate)(w1650, w1653, w1652, w1651) -> (w1654:fxp<+/-,22,10>[])
        n647 = case shown="True" "Acquire Enable" {
          tunnel: [w1659 w1662] -> w1655
          tunnel: w1656 -> [w1659 w1661]
          tunnel: w1654 -> [_ w1660]
          frame False {
          }
          frame True {
            n648 = for {
              shift-right: [w1665] -> w1662
              shift-left: w1661 -> [w1664]
              tunnel: w1660 -> [w1663] mode=indexing
              n649 = xnode ("FIFO Method Node")("Element"=w1663, "Timeout"=0) -> ("Timed Out?"=w1666:bool)  [unwired: 1 in, 1 out]
              n650 = Or(x=w1666, y=w1664) -> (x .or. y?=w1665:bool)
              "Overflow" <- w1665
            }
          }
        }
      }
      frame #9 {
        # "13. End Proc Timer"
        n651 = call "Tick Count2"() -> ("Tick Count(uSec)"=w1687:u32)
        n652 = Subtract(x=w1687, y=w1686) -> (x-y=→"Proc Time":u32)
        n653 = local read "npcountout 2"() -> (w1669:i16)
        n654 = local read "npcountout 3"() -> (w1670:i16)
        n655 = local read "npcountout 4"() -> (w1671:i16)
        n656 = local read "Hold Count 3"() -> (w1681:i16)
        n657 = local read "Hold Count 2"() -> (w1682:i16)
        n658 = local read "Hold Count 4"() -> (w1676:i16)
        n659 = local read "Hold Count 1"() -> (w1673:i16)
        n660 = local read "npcountout"() -> (w1668:i16)
        n661 = local read "Trial Live 2"() -> (w1678:bool)
        n662 = local read "Trial Live 3"() -> (w1679:bool)
        n663 = local read "Trial Live 4"() -> (w1675:bool)
        n664 = local read "Trial Live 1"() -> (w1674:bool)
        n665 = local read "Hold 3"() -> (w1680:bool)
        n666 = local read "Hold 2"() -> (w1683:bool)
        n667 = local read "Hold 4"() -> (w1677:bool)
        n668 = local read "Hold 1"() -> (w1672:bool)
      }
    }
  }
